vi "CRYGraph Property Window Wave.vi"(9 "Tab Name":string, 10 "Graph VI Ref":refnum<vi>) -> ()   [LabVIEW 2013]
uses:
  <vilib>/Utility/miscctls.llb/LVRowAndColumnTypeDef.ctl
panel:
  in  "SetFormat":bool
  in  "No Data":bool
  out "CursorStyle":string
  out "CursorPointStyle":string
  out "CursorLineWidth":string
  out "CursorLineStyle":string
  out "Scale Style":u8=5
  out "Interpolation":string
  out "PointStyle":string
  out "LineWidth":string
  out "LineStyle":string
  in  "Property Tab":T1(tab)
  in  "Background Color":u32(colorbox)
  in  "Title Name":string
  in  "Ignore timestamp information":bool
  in  "PadType":u16(ring) items=["Pad with spaces on left", "Pad with spaces on right", "Pad with zeros on left"]
  in  "Field Width":u16
  in  "Use minimum field width":bool
  in  "Exponent in multiples of 3":bool
  in  "Hide trailing zeros":bool
  in  "PrecisionDigits":u16
  in  "PrecisionType":u16(ring) items=["Digitals of precision", "Significant digits"]
  in  "Notation":i32(listbox)
  in  "FormatAxis":u16(ring) items=["X-Axis", "Y-Axis"]
  in  "TimeFormat":u16(ring) items=["Custom time format", "System time format", "Time unused"]
  in  "Digits":u16
  in  "YMD":u16(slide)
  in  "AMFM":u16(slide)=1
  in  "HMS":u16(slide)=1
  in  "DateFormat":u16(ring) items=["Custom date format", "System date format", "Date unused"]
  in  "YearShow":u16(slide)
  in  "Point/Fill":u32(colorbox)
  in  "Fill to":i16(ring) items=["none"=-1, "zero"=-2, "-Infinity"=-3, "+Infinity"=-4]
  in  "Items":u16(ring)
  out "Colors":bool
  in  "Line":u32(colorbox)
  in  "LineStyle4":bool
  in  "LineStyle3":bool
  in  "LineStyle2":bool
  in  "LineStyle0":bool
  in  "LineStyle1":bool
  in  "LineWidth5":bool
  in  "LineWidth1":bool
  in  "LineWidth4":bool
  in  "LineWidth3":bool
  in  "LineWidth2":bool
  in  "LineWidth0":bool
  in  "PointStyle16":bool
  in  "PointStyle15":bool
  in  "PointStyle14":bool
  in  "PointStyle13":bool
  in  "PointStyle12":bool
  in  "PointStyle11":bool
  in  "PointStyle10":bool
  in  "PointStyle9":bool
  in  "PointStyle8":bool
  in  "PointStyle7":bool
  in  "PointStyle6":bool
  in  "PointStyle5":bool
  in  "PointStyle4":bool
  in  "PointStyle3":bool
  in  "PointStyle2":bool
  in  "PointStyle1":bool
  in  "PointStyle0":bool
  in  "Interpolation4":bool
  in  "Interpolation5":bool
  in  "Interpolation3":bool
  in  "Interpolation2":bool
  in  "Interpolation1":bool
  in  "Interpolation0":bool
  in  "Show Plot":bool
  in  "GridStyle":u16(ring)=4
  in  "Minor grid":u32(colorbox)
  in  "Major grid":u32(colorbox)
  in  "Marker text":u32(colorbox)
  in  "Minor tick":u32(colorbox)
  in  "Major tick":u32(colorbox)
  in  "Log":bool
  in  "Show scale":bool
  in  "Show scale label":bool
  in  "Maximum":dbl
  in  "Minimum":dbl
  in  "Autoscale":bool
  in  "Axis Name":string caption="Name"
  in  "ScaleAxis":u16(ring)
  out "Grid Colors":bool
  out "Scale Style and Colors":bool
  in  "Cursor Tab":enum32{"Page 1"}(tab)
  in  "CursorPointStyle16":bool
  in  "CursorPointStyle15":bool
  in  "CursorPointStyle14":bool
  in  "CursorPointStyle13":bool
  in  "CursorPointStyle12":bool
  in  "CursorPointStyle11":bool
  in  "CursorPointStyle10":bool
  in  "CursorPointStyle9":bool
  in  "CursorPointStyle8":bool
  in  "CursorPointStyle7":bool
  in  "CursorPointStyle6":bool
  in  "CursorPointStyle5":bool
  in  "CursorPointStyle4":bool
  in  "CursorPointStyle3":bool
  in  "CursorPointStyle2":bool
  in  "CursorPointStyle1":bool
  in  "CursorPointStyle0":bool
  in  "CursorLineWidth5":bool
  in  "CursorLineWidth1":bool
  in  "CursorLineWidth4":bool
  in  "CursorLineWidth3":bool
  in  "CursorLineWidth2":bool
  in  "CursorLineWidth0":bool
  in  "CursorLineStyle4":bool
  in  "CursorLineStyle3":bool
  in  "CursorLineStyle2":bool
  in  "CursorLineStyle0":bool
  in  "CursorLineStyle1":bool
  in  "Cursor Items":u16(ring)
  in  "CursorStyle8":bool
  in  "CursorStyle4":bool
  in  "CursorStyle5":bool
  in  "CursorStyle7":bool
  in  "CursorStyle6":bool
  in  "CursorStyle3":bool
  in  "CursorStyle2":bool
  in  "CursorStyle1":bool
  in  "CursorStyle0":bool
  in  "Cursor color":u32(colorbox)
  in  "Linked to plot:":u16(ring)
  in  "Link Cursors":bool
  in  "Show Cursors":bool
  in  "OK":bool
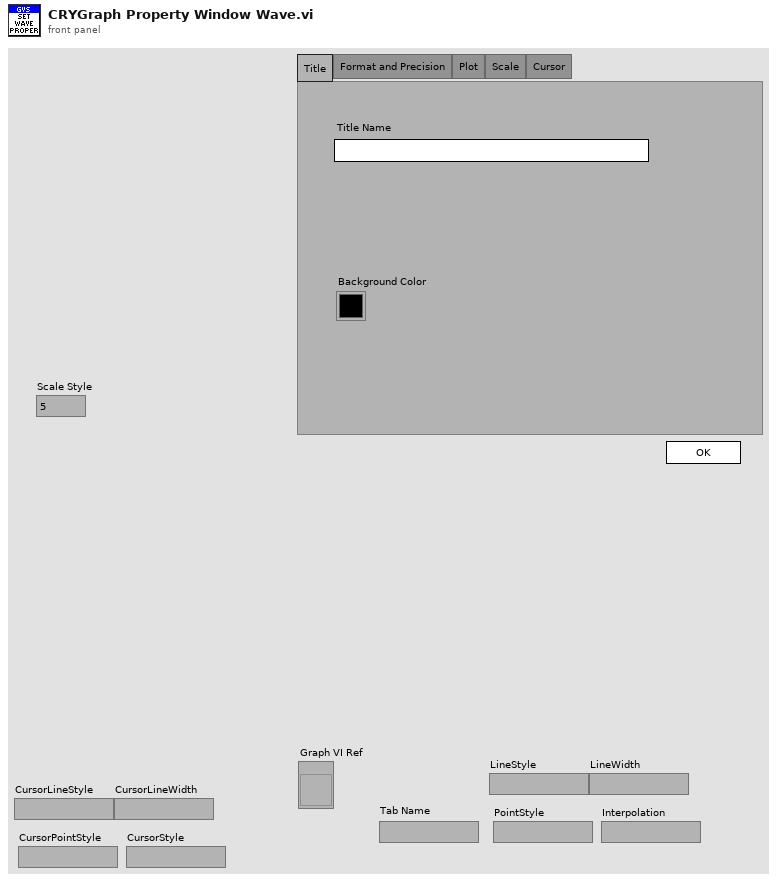
[diagram p1: front panel]
types:
  T1 = enum32{"Title", "Format and Precision", "Plots", "Scales", "Cursors"}
  T2 = enum32{"Page Enabled", "Page Disabled", "Page Disabled & Grayed"}
  T3 = enum8{"Enabled", "Disabled", "Disabled and Grayed Out"}
  T4 = typedef "LVRowAndColumnTypeDef.ctl" = cluster{"Row":i32, "Column":i32}
  T5 = typedef "CRYWaveform Cluster.ctl" = cluster{"Waveform":cluster{"X0":dbl, "dX":dbl, "Y":sgl[]}, "X data":u16, "Y data":u16, "Y axis":u16, "X unit":string, "Y unit":string, "Y dB ref":dbl, "display Y":bool, "display X":bool, "Overload?":bool, "Test Info":string, "Step No.":i32, "Name":string, "protected":bool, "Sqc history":string[], "Signal Channel ID":i32, "Plot Settings":cluster{"Color":u32, "Interpolation":u8, "Point Style":u8, "Line Style":u8, "Point Color":u32, "Line Width":u8, "Bar Plot Style":u8, "Fill To":i16}, "AutoProtect":bool}
  T6 = cluster{"Notation":i32, "PrecisionType":u16, "PrecisionDigits":u16, "Hide trailing zeros":bool, "Exponent in multiples of 3":bool, "Field Width":u16, "PadType":u16, "Use minimum field width":bool, "TimeFormat":u16, "AMFM":u16, "HMS":u16, "Digits":u16, "DateFormat":u16, "YMD":u16, "YearShow":u16}
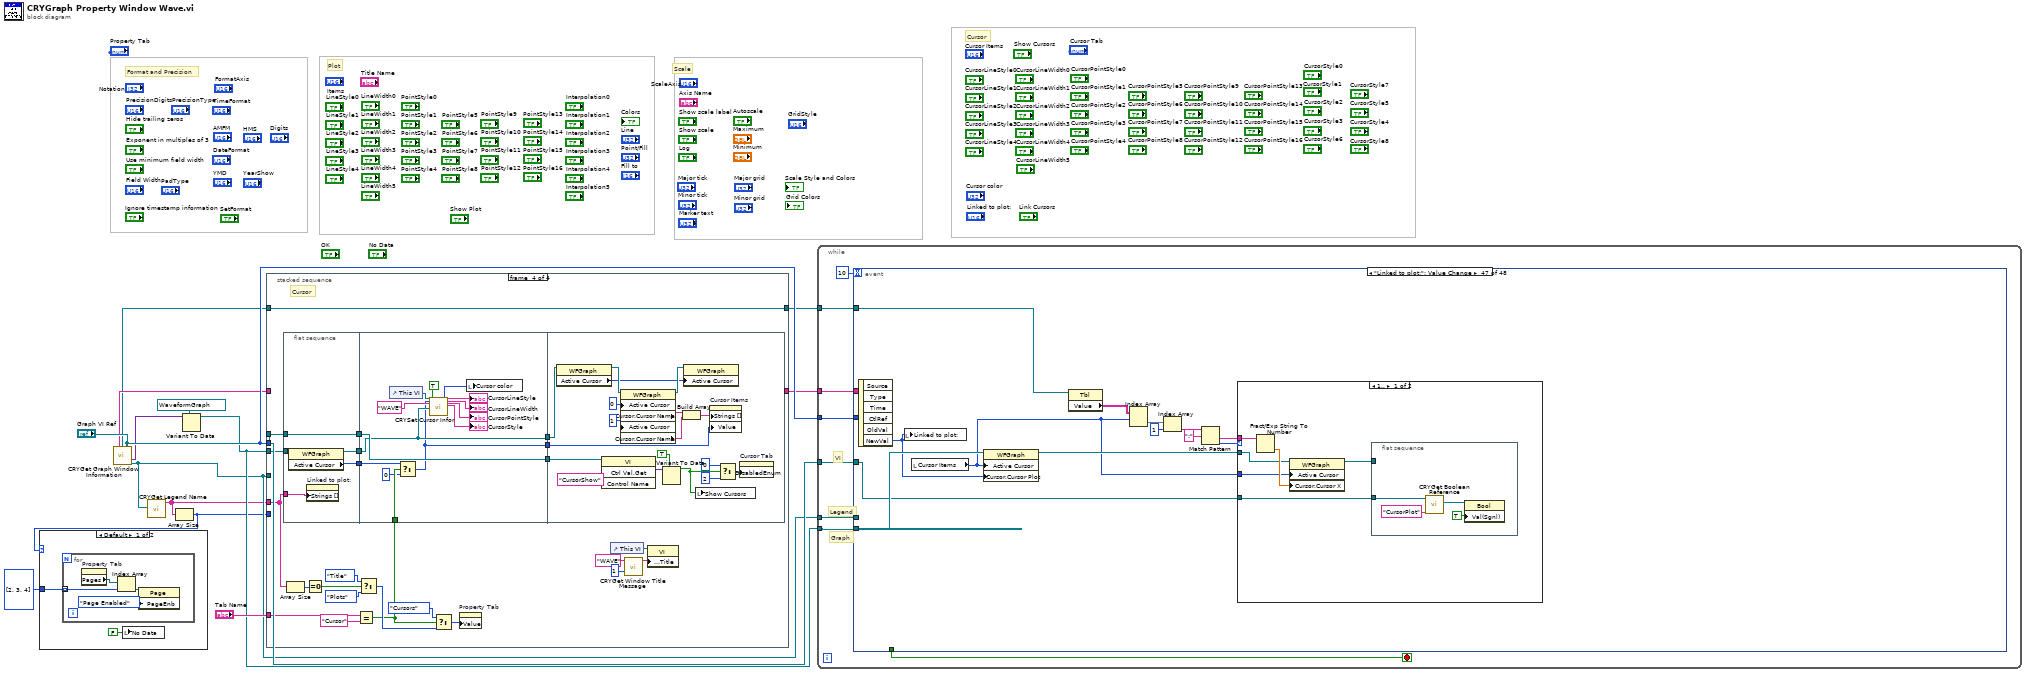
[diagram p0: block diagram]
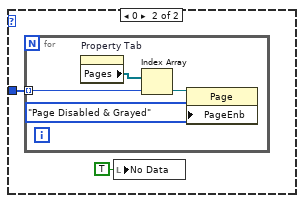
[diagram p2: hidden frame]
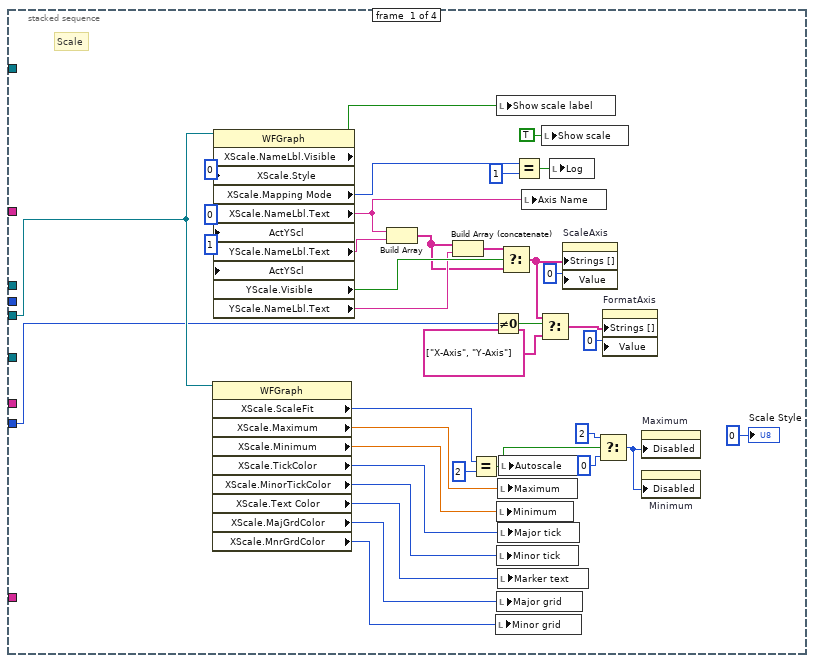
[diagram p3: hidden frame]
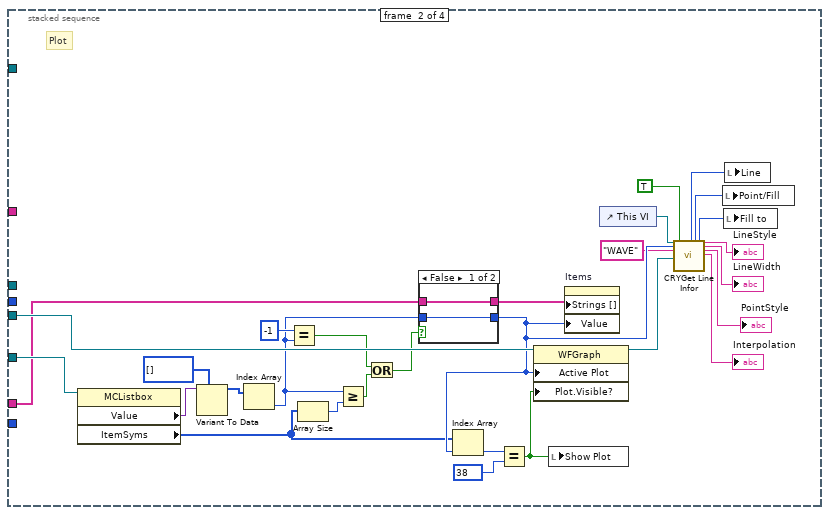
[diagram p4: hidden frame]
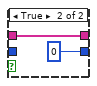
[diagram p5: hidden frame]
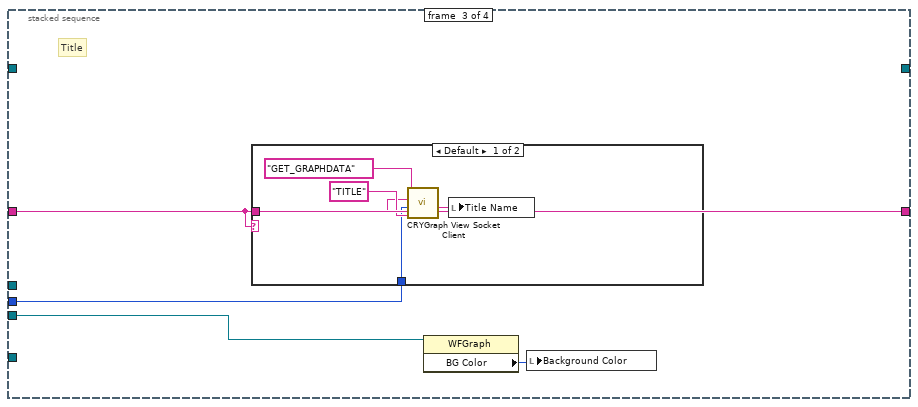
[diagram p6: hidden frame]
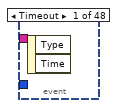
[diagram p8: hidden frame]
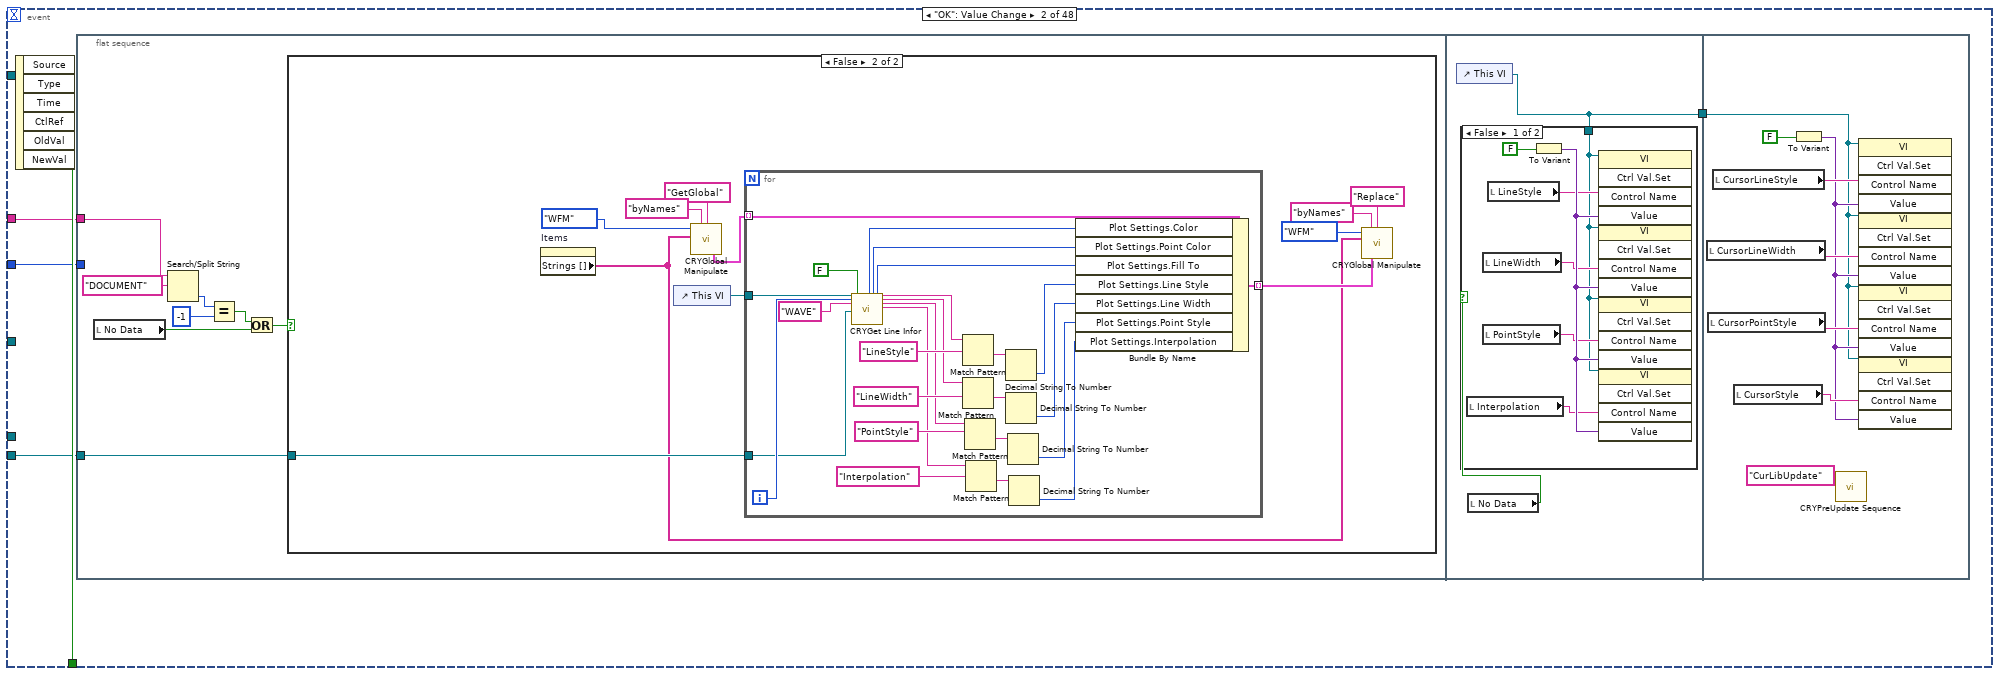
[diagram p9: hidden frame]
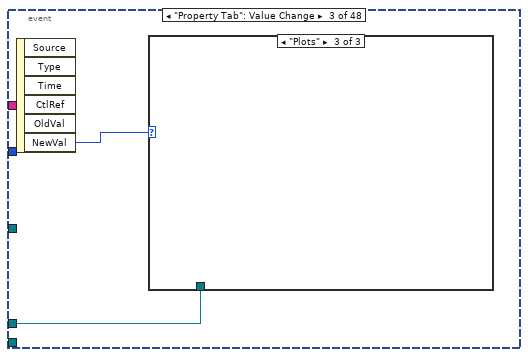
[diagram p12: hidden frame]
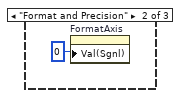
[diagram p14: hidden frame]
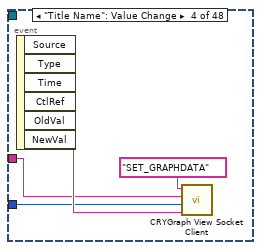
[diagram p15: hidden frame]
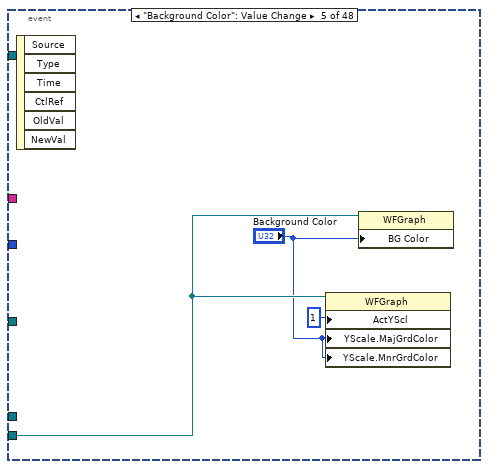
[diagram p16: hidden frame]
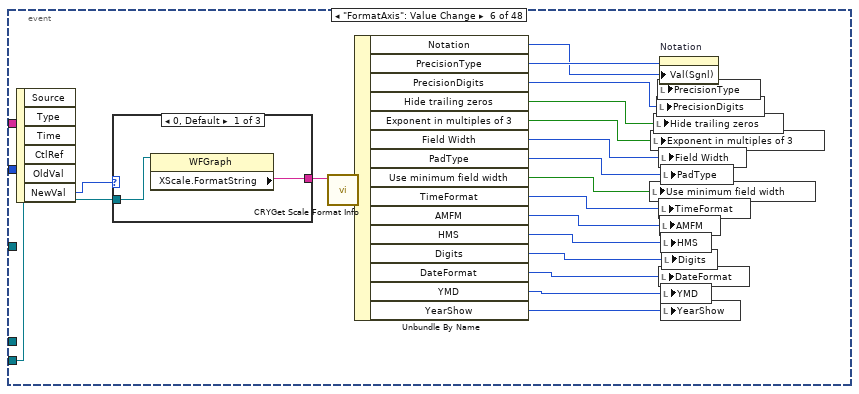
[diagram p17: hidden frame]
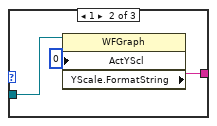
[diagram p18: hidden frame]
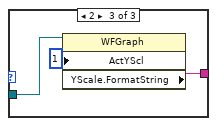
[diagram p19: hidden frame]
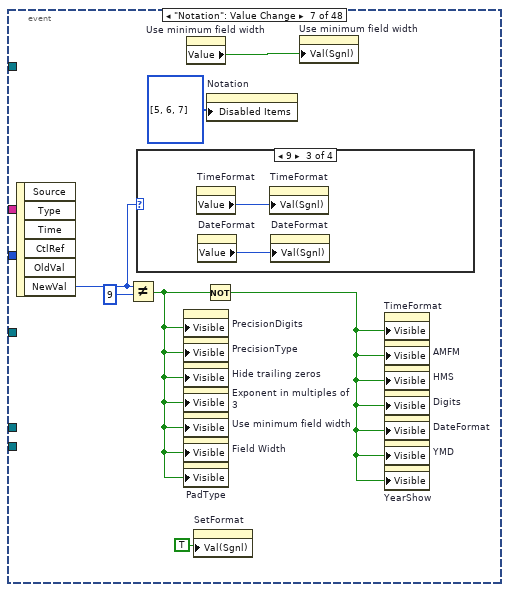
[diagram p20: hidden frame]
diagram:
  # "Format and Precision"
  # "Cursor"
  # "Scale"
  # "Plot"
  n1 = call "CRYGet Graph Window Information.vi"("pGraph VI In"="Graph VI Ref") -> ("Queue Name Out"=w10:string, "Cursor Ref Out"=w2:refnum<vi>, "Graph Number Out"=w11:i32, "Graph Control Ref Out"=w4:variant, "Legend Ref Out"=w8:refnum<vi>)  [unwired: 2 in, 8 out]
  n2 = call "CRYGet Legend Name.vi"("MCListbox Refnum"=w8) -> ("Names Out"=w7:string[])  [unwired: 1 in, 9 out]
  n3 = Array Size(array=w7) -> (size(s)=w6:i32)
  n4 = case shown="Default" w6 {
    tunnel: i32[] [2, 3, 4] -> [w15 w21]
    frame Default {
      n5 = for {
        tunnel: w15 -> [w18] mode=indexing
        n6 = property on="Property Tab" class="TabCtl (strict)"() -> ("Pages"=w17:refnum<vi>[])  [unwired: 2 in, 2 out]
        n7 = Index Array(array=w17, index=w18) -> (element=w19:refnum<vi>)
        n8 = property class="Page"(reference=w19, "PageEnb"=T2."Page Enabled" ("Page Enabled State")) -> ()  [unwired: 1 in, 2 out]
      }
      n9 = local write "No Data"(FALSE ("No Data")) -> ()
    }
    frame 0 {
      n10 = for {
        tunnel: w21 -> [w23] mode=indexing
        n11 = property on="Property Tab" class="TabCtl (strict)"() -> ("Pages"=w24:refnum<vi>[])  [unwired: 2 in, 2 out]
        n12 = Index Array(array=w24, index=w23) -> (element=w25:refnum<vi>)
        n13 = property class="Page"(reference=w25, "PageEnb"=T2."Page Disabled & Grayed" ("Page Enabled State")) -> ()  [unwired: 1 in, 2 out]
      }
      n14 = local write "No Data"(TRUE ("No Data")) -> ()
    }
  }
  n15 = Variant To Data(type=refnum<vi> refnum ("WaveGraph Ref"), Variant=w4) -> (data=w12:refnum<vi>)  [unwired: 1 in, 1 out]
  n16 = stacked-sequence {
    tunnel: w12 -> [w62 w90 w99 w128]
    tunnel: "Graph VI Ref" -> [_ _ _ w125]
    tunnel: w8 -> [_ w91 _ _]
    tunnel: "Tab Name" -> [_ _ _ w120]
    tunnel: w11 -> [_ _ w97 _]
    tunnel: w10 -> [_ _ w96 _]
    tunnel: [_ _ w96 _] -> w9
    tunnel: w7 -> [_ w89 _ w117]
    tunnel: w6 -> [w30 _ _ _]
    tunnel: w2 -> [_ _ _ w105]
    tunnel: [_ _ _ w105] -> w1
    frame #0 {
      # "Scale"
      n17 = property class="WFGraph"(reference=w62) -> ("XScale.ScaleFit"=w52:u8, "XScale.Maximum"=w51:dbl, "XScale.Minimum"=w50:dbl, "XScale.TickColor"=w43:u32, "XScale.MinorTickColor"=w42:u32, "XScale.Text Color"=w41:u32, "XScale.MajGrdColor"=w40:u32, "XScale.MnrGrdColor"=w39:u32)  [unwired: 1 in, 2 out]
      n18 = property class="WFGraph"(reference=w62, "XScale.Style"=u8 0 ("X Scale.Style"), "ActYScl"=0 ("Active Y Scale"), "ActYScl"=1 ("Active Y Scale")) -> ("XScale.NameLbl.Visible"=w59:bool, "XScale.Mapping Mode"=w55:u8, "XScale.NameLbl.Text"=w44:string, "YScale.NameLbl.Text"=w38:string, "YScale.Visible"=w36:bool, "YScale.NameLbl.Text"=w35:string)  [unwired: 1 in, 2 out]
      n19 = Build Array(w44, w38) -> (w33:string[])
      n20 = Build Array (concatenate)(w33, w35) -> (w34:string[])
      n21 = Equal?(x=w52, y=u8 2 ("X Scale.Scale Fit")) -> (x = y?=w45:bool)
      n22 = Not Equal To 0?(x=w30) -> (x != 0?=w31:bool)
      n23 = local write "Minor grid"(w39) -> ()
      n24 = local write "Show scale label"(w59) -> ()
      n25 = local write "Minimum"(w50) -> ()
      n26 = local write "Minor tick"(w42) -> ()
      n27 = local write "Major grid"(w40) -> ()
      n28 = local write "Maximum"(w51) -> ()
      n29 = local write "Major tick"(w43) -> ()
      n30 = local write "Marker text"(w41) -> ()
      n31 = local write "Autoscale"(w45) -> ()
      n32 = Select(t=w34, s=w36, f=w33) -> (s? t:f=w29:string[])
      n33 = Equal?(x=w55, y=u8 1) -> (x = y?=w56:bool)
      n34 = local write "Axis Name"(w44) -> ()
      n35 = Select(t=w29, s=w31, f=string[] ["X-Axis", "Y-Axis"]) -> (s? t:f=w28:string[])
      n36 = local write "Show scale"(TRUE ("Show scale")) -> ()
      n37 = local write "Log"(w56) -> ()
      n38 = property on="ScaleAxis" class="Ring (strict)"("Strings []"=w29, "Value"=u8 0 ("y")) -> ()  [unwired: 2 in, 2 out]
      n39 = Select(t=u8 2 ("X Scale.Scale Fit"), s=w45, f=u8 0 ("X Scale.Scale Fit")) -> (s? t:f=w47:u8)
      n40 = property on="FormatAxis" class="Ring (strict)"("Strings []"=w28, "Value"=u8 0 ("y")) -> ()  [unwired: 2 in, 2 out]
      n41 = property on="Maximum" class="DigNum (strict)"("Disabled"=w47) -> ()  [unwired: 2 in, 2 out]
      n42 = property on="Minimum" class="DigNum (strict)"("Disabled"=w47) -> ()  [unwired: 2 in, 2 out]
      "Scale Style" <- u8 0 ("X Scale.Scale Fit")
    }
    frame #1 {
      # "Plot"
      n43 = property class="MCListbox"(reference=w91) -> ("Value"=w83:variant, "ItemSyms"=w69:i32[])  [unwired: 1 in, 2 out]
      n44 = Variant To Data(type=i32[] [], Variant=w83) -> (data=w70:i32[])  [unwired: 1 in, 1 out]
      n45 = Index Array(array=w70) -> (element=w63:i32)  [unwired: 1 in]
      n46 = Equal?(x=-1, y=w63) -> (x = y?=w66:bool)
      n47 = Array Size(array=w69) -> (size(s)=w67:i32)
      n48 = Greater Or Equal?(x=w63, y=w67) -> (x >= y?=w65:bool)
      n49 = Or(x=w66, y=w65) -> (x .or. y?=w64:bool)
      n50 = case shown="False" w64 {
        tunnel: w89 -> [w93 w95]
        tunnel: [w93 w95] -> w88
        tunnel: [w92 0 ("Value")] -> w82
        tunnel: w63 -> [w92 _]
        frame False {
        }
        frame True {
        }
      }
      n51 = Index Array(array=w69, index=w82) -> (element=w86:i32)
      n52 = Equal?(x=w86, y=38) -> (x = y?=w84:bool)
      n53 = property class="WFGraph"(reference=w90, "Active Plot"=w82, "Plot.Visible?"=w84) -> (reference out=w87:refnum<vi>)  [unwired: 1 in, 1 out]
      n54 = local write "Show Plot"(w84) -> ()
      n55 = property on="Items" class="Ring (strict)"("Strings []"=w88, "Value"=w82) -> ()  [unwired: 2 in, 2 out]
      n56 = control-ref of="This VI"() -> (w77:refnum<vi>)
      n57 = call "CRYGet Line Infor.vi"("This VI"=w77, "Active Plot Number"=w82, "Graph Type"="WAVE", "Wave Graph Control Ref"=w87, "Property Set?"=TRUE) -> ("Line"=w73:u32, "Point/Fill"=w72:u32, "Fill to"=w74:i16, "LineStyle"=→"LineStyle":string, "LineWidth"=→"LineWidth":string, "PointStyle"=→"PointStyle":string, "Interpolation"=→"Interpolation":string)  [unwired: 16 in]
      n58 = local write "Point/Fill"(w72) -> ()
      n59 = local write "Fill to"(w74) -> ()
      n60 = local write "Line"(w73) -> ()
    }
    frame #2 {
      # "Title"
      n61 = case shown="Default" w96 {
        tunnel: w97 -> [w102 _]
        tunnel: w96 -> [w101 _]
        frame Default {
          n62 = call "CRYGraph View Socket Client.vi"("sOption"="TITLE", "nData"=w102, "sData"=w101, "sAction"="GET_GRAPHDATA") -> ("sData Out"=w100:string)  [unwired: 4 in, 3 out]
          n63 = local write "Title Name"(w100) -> ()
        }
        frame "test DataView" {
        }
      }
      n64 = property class="WFGraph"(reference=w99) -> ("BG Color"=w98:u32)  [unwired: 1 in, 2 out]
      n65 = local write "Background Color"(w98) -> ()
    }
    frame #3 {
      # "Cursor"
      n66 = flat-sequence {
        tunnel: w125 -> [w133]
        tunnel: w128 -> [w131]
        tunnel: [w130] -> w119
        tunnel: [w133] -> w118
        tunnel: w117 -> [w132]
        tunnel: [w129] -> w115
        tunnel: [w136] -> w127
        tunnel: [w139] -> w126
        tunnel: w119 -> [w136]
        tunnel: w118 -> [w139]
        tunnel: w116 -> [w138]
        tunnel: w115 -> [w135]
        tunnel: [w134] -> w114
        tunnel: w127 -> [w152]
        tunnel: w126 -> [w153]
        tunnel: w114 -> [w148]
        frame #0 {
          n67 = property class="WFGraph"(reference=w131) -> (reference out=w130:refnum<vi>, "Active Cursor"=w129:u32)  [unwired: 1 in, 1 out]
          n68 = property on="Linked to plot:" class="Ring (strict)"("Strings []"=w132) -> ()  [unwired: 2 in, 2 out]
        }
        frame #1 {
          n69 = control-ref of="This VI"() -> (w140:refnum<vi>)
          n70 = Select(t=w135, s=w138, f=u32 0 ("Active Cursor")) -> (s? t:f=w134:u32)
          n71 = call "CRYSet Cursor Infor.vi"("This VI"=w140, "Active Cursor"=w134, "Graph Type"="WAVE", "Wave Graph Ref"=w136, "Property Set?"=TRUE) -> ("Cursor Color"=w147:u32, "CursorLineStyle"=→"CursorLineStyle":string, "CursorLineWidth"=→"CursorLineWidth":string, "CursorPointStyle"=→"CursorPointStyle":string, "CursorStyle"=→"CursorStyle":string)  [unwired: 17 in, 1 out]
          n72 = local write "Cursor color"(w147) -> ()
        }
        frame #2 {
          n73 = property class="WFGraph"(reference=w152) -> (reference out=w151:refnum<vi>, "Active Cursor"=w149:u32)  [unwired: 1 in, 1 out]
          n74 = invoke class="VI" method="Ctrl Val.Get"(reference=w153, "Control Name"="CursorShow") -> ("Get Control Value Variant"=w158:variant)  [unwired: 2 in, 3 out]
          n75 = property class="WFGraph"(reference=w151, "Active Cursor"=u32 0, "Active Cursor"=u32 1) -> (reference out=w150:refnum<vi>, "Cursor.Cursor Name"=w163:string, "Cursor.Cursor Name"=w162:string)  [unwired: 1 in, 1 out]
          n76 = Variant To Data(type=TRUE ("Visible"), Variant=w158) -> (data=w160:bool)  [unwired: 1 in, 1 out]
          n77 = Build Array(w163, w162) -> (w161:string[])
          n78 = property class="WFGraph"(reference=w150, "Active Cursor"=w149) -> ()  [unwired: 1 in, 2 out]
          n79 = local write "Show Cursors"(w160) -> ()
          n80 = property on="Cursor Items" class="Ring (strict)"("Strings []"=w161, "Value"=w148) -> ()  [unwired: 2 in, 2 out]
          n81 = Select(t=0, s=w160, f=2) -> (s? t:f=w156:i32)
          n82 = property on="Cursor Tab" class="TabCtl (strict)"("DisabledEnum"=w156) -> ()  [unwired: 2 in, 2 out]
        }
      }
      n83 = Array Size(array=w117) -> (size(s)=w124:i32)
      n84 = Equal To 0?(x=w124) -> (x = 0?=w122:bool)
      n85 = Equal?(x=w120, y="Cursor" ("Graph Type")) -> (x = y?=w116:bool)
      n86 = Select(t=T1."Title" ("Tab Control"), s=w122, f=T1."Plots" ("Tab Control")) -> (s? t:f=w121:T1)
      n87 = Select(t=T1."Cursors" ("Tab Control"), s=w116, f=w121) -> (s? t:f=w110:T1)
      n88 = property on="Property Tab" class="TabCtl (strict)"("Value"=w110) -> ()  [unwired: 2 in, 2 out]
      n89 = control-ref of="This VI"() -> (w106:refnum<vi>)
      n90 = call "CRYGet Window Title Message.vi"("No"=1 ("Error No"), "Kind"="WAVE") -> ("Multibyte String"=w107:string)  [unwired: 4 in, 5 out]
      n91 = property class="VI"(reference=w106, "Front Panel.Title"=w107) -> ()  [unwired: 1 in, 2 out]
    }
  }
  n92 = while {
    tunnel: w12 -> [w172]
    tunnel: "Graph VI Ref" -> [w171]
    tunnel: w8 -> [w169]
    tunnel: w9 -> [w168]
    tunnel: w11 -> [w167]
    tunnel: w1 -> [w166]
    stop <- w173 stop-if-true
    # "Legend"
    # "Graph"
    # "VI"
    n93 = event shown="[46] \"Linked to plot:\": Value Change" {
      selector: _ -> [_ _ _ _ _ _ _ _ _ _ _ _ _ _ _ _ _ _ _ _ _ _ _ _ _ _ _ _ _ _ _ _ _ _ _ _ _ _ _ _ _ _ _ _ _ _ _ _]
      dyn-events: _ -> [_ _ _ _ _ _ _ _ _ _ _ _ _ _ _ _ _ _ _ _ _ _ _ _ _ _ _ _ _ _ _ _ _ _ _ _ _ _ _ _ _ _ _ _ _ _ _ _]
      timeout: 10 -> [_ _ _ _ _ _ _ _ _ _ _ _ _ _ _ _ _ _ _ _ _ _ _ _ _ _ _ _ _ _ _ _ _ _ _ _ _ _ _ _ _ _ _ _ _ _ _ _]
      tunnel: [_ w178 _ _ _ _ _ _ _ _ _ _ _ _ _ _ _ _ _ _ _ _ _ _ _ _ _ _ _ _ _ _ _ _ _ _ _ _ _ _ _ _ _ _ _ _ _ _] -> w173
      tunnel: w172 -> [_ w177 _ _ w249 w268 _ _ _ _ _ _ _ _ _ w337 w481 w513 w545 w577 w607 w640 w656 w666 w676 w704 w746 w757 w770 w786 w800 w811 w822 w833 w844 w855 w872 w928 w947 _ w971 w992 w1013 w1034 w1055 w1078 w1098 _]
      tunnel: w171 -> [_ _ _ _ _ _ _ _ _ _ _ _ _ _ _ _ _ _ _ _ _ _ _ _ _ _ _ _ _ _ _ _ _ _ _ _ w868 w925 w944 w966 _ _ _ _ _ w1079 w1086 _]
      tunnel: w169 -> [_ _ w241 _ _ _ _ _ _ _ _ _ _ _ _ _ w479 w511 w543 w575 w609 w639 w655 w663 w674 _ _ _ _ _ _ _ _ _ _ _ _ _ _ _ _ _ _ _ _ _ _ _]
      tunnel: w168 -> [_ w175 _ w245 _ _ _ _ _ _ _ _ _ _ _ _ w480 w512 w544 w576 _ _ w650 w664 w673 _ _ _ _ _ _ _ _ _ _ _ _ _ _ _ _ _ _ _ _ _ _ _]
      tunnel: w167 -> [_ w174 _ w244 _ _ _ _ _ _ _ _ _ _ _ _ _ _ _ _ _ _ _ _ _ _ _ _ _ _ _ _ _ _ _ _ _ _ _ _ _ _ _ _ _ _ _ _]
      tunnel: w166 -> [_ _ _ _ _ _ _ _ _ _ _ _ _ _ _ _ _ _ _ _ _ _ _ _ _ _ _ _ _ _ _ _ _ _ _ _ _ _ _ _ _ _ _ _ _ _ w1087 _]
      event Timeout {
        n94 = event-data() -> ()  [unwired: 3 out]
      }
      event "OK": Value Change {
        n95 = event-data() -> ("NewVal"=w178:bool)  [unwired: 6 out]
        n96 = flat-sequence {
          tunnel: w177 -> [w186]
          tunnel: w175 -> [w179]
          tunnel: w174 -> [_]
          tunnel: [w225] -> w176
          tunnel: w176 -> [w234]
          frame #0 {
            n97 = local read "No Data"() -> (w181:bool)
            n98 = Search/Split String(string=w179, search string/char (-)="DOCUMENT" ("regular expression")) -> (offset of match=w184:i32)  [unwired: 1 in, 2 out]
            n99 = Equal?(x=w184, y=-1) -> (x = y?=w182:bool)
            n100 = Or(x=w182, y=w181) -> (x .or. y?=w180:bool)
            n101 = case shown="False" w180 {
              tunnel: w186 -> [_ w197]
              frame True {
              }
              frame False {
                n102 = property on="Items" class="Ring (strict)"() -> ("Strings []"=w188:string[])  [unwired: 2 in, 2 out]
                n103 = control-ref of="This VI"() -> (w196:refnum<vi>)
                n104 = call "CRYGlobal Manipulate.vi"("Type"=enum16{"Curves", "Values", "Results", "WFM"}."WFM" ("Type In"), "sOption"="byNames", "sAction"="GetGlobal", "sData"=w188) -> ("WFM Out"=w194:T5[])  [unwired: 5 in, 6 out]
                n105 = for {
                  tunnel: w196 -> [w222]
                  tunnel: w197 -> [w204]
                  tunnel: [w199] -> w193 mode=indexing
                  tunnel: w194 -> [w198] mode=indexing
                  i -> [w206]
                  n106 = call "CRYGet Line Infor.vi"("This VI"=w222, "Active Plot Number"=w206, "Graph Type"="WAVE", "Wave Graph Control Ref"=w204, "Property Set?"=FALSE) -> ("Line"=w201:u32, "Point/Fill"=w200:u32, "Fill to"=w202:i16, "LineStyle"=w213:string, "LineWidth"=w209:string, "PointStyle"=w208:string, "Interpolation"=w207:string)  [unwired: 16 in]
                  n107 = Match Pattern(string=w213, regular expression="LineStyle") -> (after substring=w219:string)  [unwired: 4 out]
                  n108 = Match Pattern(string=w209, regular expression="LineWidth") -> (after substring=w220:string)  [unwired: 4 out]
                  n109 = Match Pattern(string=w208, regular expression="PointStyle") -> (after substring=w218:string)  [unwired: 4 out]
                  n110 = Match Pattern(string=w207, regular expression="Interpolation") -> (after substring=w215:string)  [unwired: 4 out]
                  n111 = Decimal String To Number(string=w219) -> (number=w212:i32)  [unwired: 3 out]
                  n112 = Decimal String To Number(string=w220) -> (number=w211:i32)  [unwired: 3 out]
                  n113 = Decimal String To Number(string=w218) -> (number=w210:i32)  [unwired: 3 out]
                  n114 = Decimal String To Number(string=w215) -> (number=w205:i32)  [unwired: 3 out]
                  n115 = Bundle By Name(cluster=w198, "Plot Settings.Color"=w201, "Plot Settings.Point Color"=w200, "Plot Settings.Fill To"=w202, "Plot Settings.Line Style"=w212, "Plot Settings.Line Width"=w211, "Plot Settings.Point Style"=w210, "Plot Settings.Interpolation"=w205) -> (w199:T5)
                }
                n116 = call "CRYGlobal Manipulate.vi"("Type"=enum16{"Curves", "Values", "Results", "WFM"}."WFM", "sOption"="byNames", "sAction"="Replace", "sData"=w188, "WFM"=w193) -> ()  [unwired: 4 in, 7 out]
              }
            }
          }
          frame #1 {
            n117 = control-ref of="This VI"() -> (w225:refnum<vi>)
            n118 = local read "No Data"() -> (w224:bool)
            n119 = case shown="False" w224 {
              tunnel: w225 -> [w226 _]
              frame False {
                n120 = local read "Interpolation"() -> (w227:string)
                n121 = local read "LineWidth"() -> (w229:string)
                n122 = local read "PointStyle"() -> (w228:string)
                n123 = local read "LineStyle"() -> (w230:string)
                n124 = To Variant(anything=FALSE) -> (Variant=w232:variant)
                n125 = invoke class="VI" method="Ctrl Val.Set"(reference=w226, "Control Name"=w230, "Value"=w232) -> ()  [unwired: 2 in, 5 out]
                n126 = invoke class="VI" method="Ctrl Val.Set"(reference=w226, "Control Name"=w229, "Value"=w232) -> ()  [unwired: 2 in, 5 out]
                n127 = invoke class="VI" method="Ctrl Val.Set"(reference=w226, "Control Name"=w228, "Value"=w232) -> ()  [unwired: 2 in, 5 out]
                n128 = invoke class="VI" method="Ctrl Val.Set"(reference=w226, "Control Name"=w227, "Value"=w232) -> ()  [unwired: 2 in, 5 out]
              }
              frame True {
              }
            }
          }
          frame #2 {
            n129 = local read "CursorLineWidth"() -> (w238:string)
            n130 = local read "CursorPointStyle"() -> (w239:string)
            n131 = local read "CursorLineStyle"() -> (w237:string)
            n132 = local read "CursorStyle"() -> (w240:string)
            n133 = To Variant(anything=FALSE) -> (Variant=w235:variant)
            n134 = call "CRYPreUpdate Sequence.vi"("EventName"="CurLibUpdate") -> ()  [unwired: 15 in]
            n135 = invoke class="VI" method="Ctrl Val.Set"(reference=w234, "Control Name"=w237, "Value"=w235) -> ()  [unwired: 2 in, 5 out]
            n136 = invoke class="VI" method="Ctrl Val.Set"(reference=w234, "Control Name"=w238, "Value"=w235) -> ()  [unwired: 2 in, 5 out]
            n137 = invoke class="VI" method="Ctrl Val.Set"(reference=w234, "Control Name"=w239, "Value"=w235) -> ()  [unwired: 2 in, 5 out]
            n138 = invoke class="VI" method="Ctrl Val.Set"(reference=w234, "Control Name"=w240, "Value"=w235) -> ()  [unwired: 2 in, 5 out]
          }
        }
      }
      event "Property Tab": Value Change {
        n139 = event-data() -> ("NewVal"=w242:T1)  [unwired: 6 out]
        n140 = case shown="\"Plots\"" w242 {
          tunnel: w241 -> [_ _ _]
          frame "Title", Default {
          }
          frame "Format and Precision" {
            n141 = property on="FormatAxis" class="Ring (strict)"("Val(Sgnl)"=0 ("Value (Signaling)")) -> ()  [unwired: 2 in, 2 out]
          }
          frame "Plots" {
          }
        }
      }
      event "Title Name": Value Change {
        n142 = event-data() -> ("NewVal"=w246:string)  [unwired: 6 out]
        n143 = call "CRYGraph View Socket Client.vi"("sOption"=w246, "nData"=w244, "sData"=w245, "sAction"="SET_GRAPHDATA") -> ()  [unwired: 4 in, 4 out]
      }
      event "Background Color": Value Change {
        n144 = event-data() -> ()  [unwired: 7 out]
        n145 = property on="Property Node" class="WFGraph"(reference=w249, "ActYScl"=1 ("Active Y Scale"), "YScale.MajGrdColor"="Background Color", "YScale.MnrGrdColor"="Background Color") -> ()  [unwired: 1 in, 2 out]
        n146 = property class="WFGraph"(reference=w249, "BG Color"="Background Color") -> ()  [unwired: 1 in, 2 out]
      }
      event "FormatAxis": Value Change {
        n147 = event-data() -> ("NewVal"=w269:u16)  [unwired: 6 out]
        n148 = case shown="0, Default" w269 {
          tunnel: w268 -> [w271 w274 w277]
          tunnel: [w270 w272 w275] -> w267
          frame 0, Default {
            n149 = property class="WFGraph"(reference=w271) -> ("XScale.FormatString"=w270:string)  [unwired: 1 in, 2 out]
          }
          frame 1 {
            n150 = property class="WFGraph"(reference=w274, "ActYScl"=0 ("Active Y Scale")) -> ("YScale.FormatString"=w272:string)  [unwired: 1 in, 2 out]
          }
          frame 2 {
            n151 = property class="WFGraph"(reference=w277, "ActYScl"=1 ("Active Y Scale")) -> ("YScale.FormatString"=w275:string)  [unwired: 1 in, 2 out]
          }
        }
        n152 = call "CRYGet Scale Format Info.vi"("FormatString"=w267) -> ("ScaleFormat"=w266:T6)  [unwired: 10 in]
        n153 = Unbundle By Name(w266) -> ("Notation"=w259:i32, "PrecisionType"=w265:u16, "PrecisionDigits"=w264:u16, "Hide trailing zeros"=w263:bool, "Exponent in multiples of 3"=w262:bool, "Field Width"=w261:u16, "PadType"=w260:u16, "Use minimum field width"=w258:bool, "TimeFormat"=w257:u16, "AMFM"=w256:u16, "HMS"=w255:u16, "Digits"=w254:u16, "DateFormat"=w253:u16, "YMD"=w252:u16, "YearShow"=w251:u16)
        n154 = local write "Use minimum field width"(w258) -> ()
        n155 = local write "Exponent in multiples of 3"(w262) -> ()
        n156 = local write "Hide trailing zeros"(w263) -> ()
        n157 = local write "PrecisionDigits"(w264) -> ()
        n158 = local write "PrecisionType"(w265) -> ()
        n159 = local write "Field Width"(w261) -> ()
        n160 = local write "TimeFormat"(w257) -> ()
        n161 = local write "DateFormat"(w253) -> ()
        n162 = property on="Notation" class="LstBox (strict)"("Val(Sgnl)"=w259) -> ()  [unwired: 2 in, 2 out]
        n163 = local write "AMFM"(w256) -> ()
        n164 = local write "PadType"(w260) -> ()
        n165 = local write "HMS"(w255) -> ()
        n166 = local write "YMD"(w252) -> ()
        n167 = local write "YearShow"(w251) -> ()
        n168 = local write "Digits"(w254) -> ()
      }
      event "Notation": Value Change {
        n169 = event-data() -> ("NewVal"=w283:i32)  [unwired: 6 out]
        n170 = Not Equal?(x=w283, y=9) -> (x != y?=w281:bool)
        n171 = case shown="9" w283 {
          frame 0, 3 {
            n172 = property on="Exponent in multiples of 3" class="Bool (strict)"("DisabledEnum"=T3."Enabled" ("Disabled")) -> ()  [unwired: 2 in, 2 out]
          }
          frame 1, 2 {
            n173 = property on="Exponent in multiples of 3" class="Bool (strict)"("DisabledEnum"=T3."Disabled and Grayed Out" ("Disabled")) -> ()  [unwired: 2 in, 2 out]
          }
          frame 9 {
            n174 = property on="TimeFormat" class="Ring (strict)"() -> ("Value"=w288:u16)  [unwired: 2 in, 2 out]
            n175 = property on="DateFormat" class="Ring (strict)"() -> ("Value"=w287:u16)  [unwired: 2 in, 2 out]
            n176 = property on="TimeFormat" class="Ring (strict)"("Val(Sgnl)"=w288) -> ()  [unwired: 2 in, 2 out]
            n177 = property on="DateFormat" class="Ring (strict)"("Val(Sgnl)"=w287) -> ()  [unwired: 2 in, 2 out]
          }
          frame Default {
          }
        }
        n178 = property on="PrecisionDigits" class="DigNum (strict)"("Visible"=w281) -> ()  [unwired: 2 in, 2 out]
        n179 = property on="PrecisionType" class="Ring (strict)"("Visible"=w281) -> ()  [unwired: 2 in, 2 out]
        n180 = property on="Hide trailing zeros" class="Bool (strict)"("Visible"=w281) -> ()  [unwired: 2 in, 2 out]
        n181 = property on="Exponent in multiples of 3" class="Bool (strict)"("Visible"=w281) -> ()  [unwired: 2 in, 2 out]
        n182 = property on="Use minimum field width" class="Bool (strict)"("Visible"=w281) -> ()  [unwired: 2 in, 2 out]
        n183 = property on="Field Width" class="DigNum (strict)"("Visible"=w281) -> ()  [unwired: 2 in, 2 out]
        n184 = property on="PadType" class="Ring (strict)"("Visible"=w281) -> ()  [unwired: 2 in, 2 out]
        n185 = property on="Use minimum field width" class="Bool (strict)"() -> ("Value"=w278:bool)  [unwired: 2 in, 2 out]
        n186 = property on="SetFormat" class="Bool (strict)"("Val(Sgnl)"=TRUE ("Value (Signaling)")) -> ()  [unwired: 2 in, 2 out]
        n187 = Not(x=w281) -> (.not. x?=w280:bool)
        n188 = property on="Notation" class="LstBox (strict)"("Disabled Items"=i32[] [5, 6, 7]) -> ()  [unwired: 2 in, 2 out]
        n189 = property on="Use minimum field width" class="Bool (strict)"("Val(Sgnl)"=w278) -> ()  [unwired: 2 in, 2 out]
        n190 = property on="TimeFormat" class="Ring (strict)"("Visible"=w280) -> ()  [unwired: 2 in, 2 out]
        n191 = property on="AMFM" class="Slide (strict)"("Visible"=w280) -> ()  [unwired: 2 in, 2 out]
        n192 = property on="HMS" class="Slide (strict)"("Visible"=w280) -> ()  [unwired: 2 in, 2 out]
        n193 = property on="Digits" class="DigNum (strict)"("Visible"=w280) -> ()  [unwired: 2 in, 2 out]
        n194 = property on="DateFormat" class="Ring (strict)"("Visible"=w280) -> ()  [unwired: 2 in, 2 out]
        n195 = property on="YMD" class="Slide (strict)"("Visible"=w280) -> ()  [unwired: 2 in, 2 out]
        n196 = property on="YearShow" class="Slide (strict)"("Visible"=w280) -> ()  [unwired: 2 in, 2 out]
      }
      event "PrecisionType", "PrecisionDigits", "Hide trailing zeros", "Exponent in multiples of 3", "PadType": Value Change {
        n197 = event-data() -> ()  [unwired: 7 out]
        n198 = property on="SetFormat" class="Bool (strict)"("Val(Sgnl)"=TRUE ("Value (Signaling)")) -> ()  [unwired: 2 in, 2 out]
      }
      event "Use minimum field width": Value Change {
        n199 = event-data() -> ("NewVal"=w298:bool)  [unwired: 6 out]
        n200 = property on="Field Width" class="DigNum (strict)"() -> ("Value"=w291:u16)  [unwired: 2 in, 2 out]
        n201 = Equal To 0?(x=w291) -> (x = 0?=w293:bool)
        n202 = Select(t=u16 1 ("Field Width"), s=w293, f=w291) -> (s? t:f=w290:u16)
        n203 = Select(t=T3."Enabled" ("Disabled"), s=w298, f=T3."Disabled and Grayed Out") -> (s? t:f=w299:T3)
        n204 = Select(t=w290, s=w298, f=u16 0 ("Field Width")) -> (s? t:f=w296:u16)
        n205 = property on="Field Width" class="DigNum (strict)"("DisabledEnum"=w299) -> ()  [unwired: 2 in, 2 out]
        n206 = property on="PadType" class="Ring (strict)"("DisabledEnum"=w299) -> ()  [unwired: 2 in, 2 out]
        n207 = property on="Field Width" class="DigNum (strict)"("Value"=w296) -> (error out=w294:errorcluster)  [unwired: 2 in, 1 out]
        n208 = property on="SetFormat" class="Bool (strict)"(error in=w294, "Val(Sgnl)"=TRUE ("Value (Signaling)")) -> ()  [unwired: 1 in, 2 out]
      }
      event "Field Width": Value Change {
        n209 = event-data() -> ("NewVal"=w309:u16)  [unwired: 6 out]
        n210 = property on="SetFormat" class="Bool (strict)"("Val(Sgnl)"=TRUE ("Value (Signaling)")) -> ()  [unwired: 2 in, 2 out]
        n211 = Equal To 0?(x=w309) -> (x = 0?=w305:bool)
        n212 = Select(t=T3."Disabled and Grayed Out" ("Disabled"), s=w305, f=T3."Enabled" ("Disabled")) -> (s? t:f=w306:T3)
        n213 = Select(t=FALSE ("x = 0?"), s=w305, f=TRUE ("x = 0?")) -> (s? t:f=w302:bool)
        n214 = property on="PadType" class="Ring (strict)"("DisabledEnum"=w306) -> ()  [unwired: 2 in, 2 out]
        n215 = property on="Field Width" class="DigNum (strict)"("DisabledEnum"=w306) -> ()  [unwired: 2 in, 2 out]
        n216 = local write "Use minimum field width"(w302) -> ()
      }
      event "TimeFormat": Value Change {
        n217 = event-data() -> ("NewVal"=w314:u16)  [unwired: 6 out]
        n218 = property on="SetFormat" class="Bool (strict)"("Val(Sgnl)"=TRUE ("Value (Signaling)")) -> ()  [unwired: 2 in, 2 out]
        n219 = case shown="0, Default" w314 {
          tunnel: [T3."Enabled" ("Disabled") T3."Disabled and Grayed Out" ("Disabled") T3."Disabled and Grayed Out" ("Disabled")] -> w313
          tunnel: [T3."Enabled" ("Disabled") T3."Enabled" ("Disabled") T3."Disabled and Grayed Out" ("Disabled")] -> w312
          frame 0, Default {
            n220 = property on="HMS" class="Slide (strict)"() -> ("Value"=w315:u16)  [unwired: 2 in, 2 out]
            n221 = property on="HMS" class="Slide (strict)"("Val(Sgnl)"=w315) -> ()  [unwired: 2 in, 2 out]
          }
          frame 1 {
          }
          frame 2 {
          }
        }
        n222 = property on="AMFM" class="Slide (strict)"("DisabledEnum"=w313) -> ()  [unwired: 2 in, 2 out]
        n223 = property on="HMS" class="Slide (strict)"("DisabledEnum"=w313) -> ()  [unwired: 2 in, 2 out]
        n224 = property on="Digits" class="DigNum (strict)"("DisabledEnum"=w312) -> ()  [unwired: 2 in, 2 out]
      }
      event "AMFM", "Digits", "YMD", "YearShow": Value Change {
        n225 = event-data() -> ()  [unwired: 7 out]
        n226 = property on="SetFormat" class="Bool (strict)"("Val(Sgnl)"=TRUE ("Value (Signaling)")) -> ()  [unwired: 2 in, 2 out]
      }
      event "HMS": Value Change {
        n227 = event-data() -> ("NewVal"=w328:u16)  [unwired: 6 out]
        n228 = property on="SetFormat" class="Bool (strict)"("Val(Sgnl)"=TRUE ("Value (Signaling)")) -> ()  [unwired: 2 in, 2 out]
        n229 = Equal To 0?(x=w328) -> (x = 0?=w327:bool)
        n230 = Select(t=T3."Disabled and Grayed Out" ("Disabled"), s=w327, f=T3."Enabled" ("Disabled")) -> (s? t:f=w324:T3)
        n231 = property on="Digits" class="DigNum (strict)"("DisabledEnum"=w324) -> ()  [unwired: 2 in, 2 out]
      }
      event "DateFormat": Value Change {
        n232 = event-data() -> ("NewVal"=w331:u16)  [unwired: 6 out]
        n233 = case shown="1, 2" w331 {
          tunnel: [T3."Enabled" ("Disabled") T3."Disabled and Grayed Out" ("Disabled")] -> w330
          frame 0, Default {
          }
          frame 1, 2 {
          }
        }
        n234 = property on="SetFormat" class="Bool (strict)"("Val(Sgnl)"=TRUE ("Value (Signaling)")) -> ()  [unwired: 2 in, 2 out]
        n235 = property on="YearShow" class="Slide (strict)"("DisabledEnum"=w330) -> ()  [unwired: 2 in, 2 out]
        n236 = property on="YMD" class="Slide (strict)"("DisabledEnum"=w330) -> ()  [unwired: 2 in, 2 out]
      }
      event "Ignore timestamp information": Value Change {
        n237 = event-data() -> ()  [unwired: 7 out]
        n238 = property on="SetFormat" class="Bool (strict)"("Val(Sgnl)"=TRUE ("Value (Signaling)")) -> ()  [unwired: 2 in, 2 out]
      }
      event "SetFormat": Value Change {
        n239 = event-data() -> ()  [unwired: 7 out]
        n240 = local read "Notation"() -> (w335:i32)
        n241 = case shown="0..3, 5..7, Default" w335 {
          tunnel: w335 -> [w348 _]
          tunnel: [w341 w380] -> w336
          frame 0..3, 5..7, Default {
            # "%[$][-][+][#][^][0][Width][.Precision || _SignificantDigits][{Unit}][<Embedded information>]Conversion"
            n242 = local read "Exponent in multiples of 3"() -> (w344:bool)
            n243 = local read "Use minimum field width"() -> (w342:bool)
            n244 = local read "Hide trailing zeros"() -> (w345:bool)
            n245 = local read "PrecisionDigits"() -> (w340:u16)
            n246 = local read "PrecisionType"() -> (w346:u16)
            n247 = local read "Field Width"() -> (w343:u16)
            n248 = local read "PadType"() -> (w347:u16)
            n249 = Select(t="#" ("format string"), s=w345, f="" ("format string")) -> (s? t:f=w357:string)
            n250 = Select(t="^" ("format string"), s=w344, f="" ("format string")) -> (s? t:f=w360:string)
            n251 = case shown="True" w342 {
              tunnel: w347 -> [_ w374]
              tunnel: w343 -> [_ w369]
              tunnel: [w366 w373] -> w362
              tunnel: [w366 w367] -> w363
              tunnel: [w366 w372] -> w361
              frame False {
                w366 = ""
              }
              frame True {
                n252 = Not Equal To 0?(x=w369) -> (x != 0?=w370:bool)
                n253 = case shown="2" w374 {
                  tunnel: [w375 "" ("format string") "0" ("format string")] -> w373
                  tunnel: [w375 "-" ("format string") "" ("format string")] -> w372
                  frame 0, Default {
                    w375 = "" ("format string")
                  }
                  frame 1 {
                  }
                  frame 2 {
                  }
                }
                n254 = Number To Decimal String(number=w369) -> (decimal integer string=w368:string)  [unwired: 1 in]
                n255 = Select(t=w368, s=w370, f="") -> (s? t:f=w367:string)
              }
            }
            n256 = Number To Decimal String(number=w340) -> (decimal integer string=w339:string)  [unwired: 1 in]
            n257 = Equal?(x=w346, y=u16 0) -> (x = y?=w354:bool)
            n258 = Index Array(array=string[] ["f", "e", "g", "p", "", "x", "o", "b", "", "T"], index=w348) -> (element=w365:string)
            n259 = Select(t="." ("format string"), s=w354, f="_" ("format string")) -> (s? t:f=w364:string)
            n260 = Concatenate Strings("%" ("string"), w361, w357, w360, w362, w363, w364, w339, w365) -> (w341:string)
          }
          frame 9 {
            n261 = local read "DateFormat"() -> (w402:u16)
            n262 = local read "TimeFormat"() -> (w398:u16)
            n263 = local read "YearShow"() -> (w404:u16)
            n264 = local read "AMFM"() -> (w399:u16)
            n265 = local read "Digits"() -> (w401:u16)
            n266 = local read "HMS"() -> (w400:u16)
            n267 = local read "YMD"() -> (w403:u16)
            n268 = Equal?(x=w402, y=u16 2) -> (x = y?=w395:bool)
            n269 = Equal?(x=w398, y=u16 2) -> (x = y?=w394:bool)
            n270 = case shown="0, Default" w398 {
              tunnel: w399 -> [w461 _ _]
              tunnel: w400 -> [w459 _ _]
              tunnel: w401 -> [w445 w463 _]
              tunnel: [w448 w462 w465] -> w381
              tunnel: w402 -> [_ _ w470]
              frame 0, Default {
                # "Custom Format"
                n271 = Equal To 0?(x=w461) -> (x = 0?=w452:bool)
                n272 = Not Equal To 0?(x=w445) -> (x != 0?=w447:bool)
                n273 = Equal To 0?(x=w459) -> (x = 0?=w456:bool)
                n274 = Format Into String(format string=":%%S%%%du", w445) -> (resulting string=w444:string)  [unwired: 2 in, 1 out]
                n275 = Select(t="%I:%M" ("format string"), s=w452, f="%H:%M" ("format string")) -> (s? t:f=w457:string)
                n276 = Select(t=w444, s=w447, f=":%S" ("format string")) -> (s? t:f=w443:string)
                n277 = Select(t="", s=w456, f=w443) -> (s? t:f=w453:string)
                n278 = Select(t=" %p", s=w452, f="" ("t")) -> (s? t:f=w449:string)
                n279 = Concatenate Strings(w457, w453, w449) -> (w448:string)
              }
              frame 1 {
                # "System Format"
                n280 = Format Into String(format string="%%.%dX", w463) -> (resulting string=w462:string)  [unwired: 2 in, 1 out]
              }
              frame 2 {
                # "No Used"
                n281 = Equal?(x=w470, y=u16 2) -> (x = y?=w468:bool)
                n282 = Select(t="%.3X" ("format string"), s=w468, f="") -> (s? t:f=w465:string)
              }
            }
            n283 = case shown="0, Default" w402 {
              tunnel: w403 -> [w411 _ _]
              tunnel: w404 -> [w410 _ _]
              tunnel: [w408 "%x" ("format string") w437] -> w382
              tunnel: w398 -> [_ _ w438]
              frame 0, Default {
                # "Custom Format"
                n284 = case shown="2" w410 {
                  tunnel: ["" ("format string") "%y" ("format string") "%Y" ("format string")] -> w409
                  frame 0, Default {
                  }
                  frame 1 {
                  }
                  frame 2 {
                  }
                }
                n285 = case shown="2" w411 {
                  tunnel: w409 -> [w416 w423 w431]
                  tunnel: [w420 w427 w435] -> w408
                  frame 0, Default {
                    n286 = Empty String/Path?(string/path=w416) -> (empty?=w419:bool)
                    n287 = Concatenate Strings("/" ("string"), w416) -> (w417:string)
                    n288 = Select(t=w416, s=w419, f=w417) -> (s? t:f=w418:string)
                    n289 = Concatenate Strings("%m/%d" ("format string"), w418) -> (w420:string)
                  }
                  frame 1 {
                    n290 = Empty String/Path?(string/path=w423) -> (empty?=w426:bool)
                    n291 = Concatenate Strings("/" ("string"), w423) -> (w424:string)
                    n292 = Select(t=w423, s=w426, f=w424) -> (s? t:f=w425:string)
                    n293 = Concatenate Strings("%d/%m" ("format string"), w425) -> (w427:string)
                  }
                  frame 2 {
                    n294 = Empty String/Path?(string/path=w431) -> (empty?=w434:bool)
                    n295 = Concatenate Strings(w431, "/" ("string")) -> (w433:string)
                    n296 = Select(t=w431, s=w434, f=w433) -> (s? t:f=w430:string)
                    n297 = Concatenate Strings(w430, "%m/%d" ("format string")) -> (w435:string)
                  }
                }
              }
              frame 1 {
                # "System Format"
              }
              frame 2 {
                # "No Used"
                n298 = Equal?(x=w438, y=u16 2) -> (x = y?=w440:bool)
                n299 = Select(t="%x" ("format string"), s=w440, f="") -> (s? t:f=w437:string)
              }
            }
            n300 = Compound Arithmetic op=AND(w395, w394) -> (w387:bool)
            n301 = Compound Arithmetic op=AND(invert w395, w394) -> (w391:bool)
            n302 = Compound Arithmetic op=AND(w395, invert w394) -> (w392:bool)
            n303 = Compound Arithmetic op=AND(invert w395, invert w394) -> (w396:bool)
            n304 = Compound Arithmetic op=OR(w391, w392) -> (w393:bool)
            n305 = Build Array(w387, w393, w396) -> (w388:bool[])
            n306 = Search 1D Array(1D array=w388, element=TRUE) -> (index of element=w390:i32)  [unwired: 1 in]
            n307 = case shown="2" w390 {
              tunnel: [" " ("format string") "" ("format string") "\n" ("format string")] -> w397
              frame 0, Default {
              }
              frame 1 {
              }
              frame 2 {
              }
            }
            n308 = Concatenate Strings("%<" ("string"), w381, w397, w382, ">T" ("string")) -> (w380:string)
          }
        }
        n309 = local read "FormatAxis"() -> (w338:u16)
        n310 = case shown="0, Default" w338 {
          tunnel: w337 -> [w472 w475 w478]
          tunnel: w336 -> [w471 w473 w476]
          frame 0, Default {
            n311 = property class="WFGraph"(reference=w472, "XScale.FormatString"=w471) -> ()  [unwired: 1 in, 2 out]
          }
          frame 1 {
            n312 = property class="WFGraph"(reference=w475, "ActYScl"=0 ("Active Y Scale"), "YScale.FormatString"=w473) -> ()  [unwired: 1 in, 2 out]
          }
          frame 2 {
            n313 = property class="WFGraph"(reference=w478, "ActYScl"=1 ("Active Y Scale"), "YScale.FormatString"=w476) -> ()  [unwired: 1 in, 2 out]
          }
        }
      }
      event "LineStyle0", "LineStyle1", "LineStyle2", "LineStyle3", "LineStyle4": Value Change {
        n314 = event-data() -> ("CtlRef"=w485:refnum<vi>)  [unwired: 6 out]
        n315 = property class="Bool (strict)"(reference=w485) -> ("Label.Text"=w483:string)  [unwired: 1 in, 2 out]
        n316 = local read "LineStyle"() -> (w482:string)
        n317 = Equal?(x=w483, y=w482) -> (x = y?=w484:bool)
        n318 = case shown="False" w484 {
          tunnel: w483 -> [w494 w507]
          tunnel: w482 -> [w500 _]
          tunnel: w481 -> [w490 _]
          tunnel: w480 -> [w488 _]
          tunnel: w479 -> [w487 _]
          frame False {
            n319 = control-ref of="This VI"() -> (w501:refnum<vi>)
            n320 = Match Pattern(string=w494, regular expression="LineStyle") -> (after substring=w492:string)  [unwired: 4 out]
            n321 = To Variant(anything=TRUE) -> (Variant=w498:variant)
            n322 = Decimal String To Number(string=w492) -> (number=w491:i32)  [unwired: 3 out]
            n323 = invoke class="VI" method="Ctrl Val.Set"(reference=w501, "Control Name"=w494, "Value"=w498) -> (reference out=w499:refnum<vi>)  [unwired: 2 in, 4 out]
            n324 = To Unsigned Byte Integer(number=w491) -> (unsigned 8bit integer=w486:u8)
            n325 = local write "LineStyle"(w494) -> ()
            n326 = To Variant(anything=FALSE) -> (Variant=w496:variant)
            n327 = property class="WFGraph"(reference=w490, "Plot.Line Style"=w486) -> ()  [unwired: 1 in, 2 out]
            n328 = invoke class="VI" method="Ctrl Val.Set"(reference=w499, "Control Name"=w500, "Value"=w496) -> ()  [unwired: 2 in, 5 out]
            n329 = property on="Items" class="Ring (strict)"() -> ("Value"=w489:u16)  [unwired: 2 in, 2 out]
            n330 = case shown="Default" w488 {
              tunnel: w487 -> [_ w505]
              tunnel: w486 -> [_ w502]
              tunnel: w489 -> [_ w504]
              frame "ViewReport" {
              }
              frame Default {
                n331 = call "CRYSet Plot Settings.vi"("Style"=w502, "sAction"="LineStyle", "Row"=w504, "Legend Refnum"=w505, "Type"=enum16{"Curves", "Values", "Results", "WFM"}."WFM") -> ()  [unwired: 2 in, 5 out]
              }
            }
          }
          frame True {
            n332 = control-ref of="This VI"() -> (w510:refnum<vi>)
            n333 = To Variant(anything=TRUE) -> (Variant=w509:variant)
            n334 = invoke class="VI" method="Ctrl Val.Set"(reference=w510, "Control Name"=w507, "Value"=w509) -> ()  [unwired: 2 in, 5 out]
          }
        }
      }
      event "LineWidth0", "LineWidth1", "LineWidth2", "LineWidth3", "LineWidth4", "LineWidth5": Value Change {
        n335 = event-data() -> ("CtlRef"=w514:refnum<vi>)  [unwired: 6 out]
        n336 = property class="Bool (strict)"(reference=w514) -> ("Label.Text"=w516:string)  [unwired: 1 in, 2 out]
        n337 = local read "LineWidth"() -> (w515:string)
        n338 = Equal?(x=w516, y=w515) -> (x = y?=w517:bool)
        n339 = case shown="False" w517 {
          tunnel: w516 -> [w524 w539]
          tunnel: w515 -> [w532 _]
          tunnel: w513 -> [w522 _]
          tunnel: w512 -> [w520 _]
          tunnel: w511 -> [w519 _]
          frame False {
            n340 = control-ref of="This VI"() -> (w533:refnum<vi>)
            n341 = Match Pattern(string=w524, regular expression="LineWidth") -> (after substring=w525:string)  [unwired: 4 out]
            n342 = To Variant(anything=TRUE) -> (Variant=w530:variant)
            n343 = Decimal String To Number(string=w525) -> (number=w526:i32)  [unwired: 3 out]
            n344 = invoke class="VI" method="Ctrl Val.Set"(reference=w533, "Control Name"=w524, "Value"=w530) -> (reference out=w531:refnum<vi>)  [unwired: 2 in, 4 out]
            n345 = To Unsigned Byte Integer(number=w526) -> (unsigned 8bit integer=w518:u8)
            n346 = local write "LineWidth"(w524) -> ()
            n347 = To Variant(anything=FALSE) -> (Variant=w528:variant)
            n348 = property class="WFGraph"(reference=w522, "Plot.Line Width"=w518) -> ()  [unwired: 1 in, 2 out]
            n349 = invoke class="VI" method="Ctrl Val.Set"(reference=w531, "Control Name"=w532, "Value"=w528) -> ()  [unwired: 2 in, 5 out]
            n350 = property on="Items" class="Ring (strict)"() -> ("Value"=w521:u16)  [unwired: 2 in, 2 out]
            n351 = case shown="Default" w520 {
              tunnel: w519 -> [_ w537]
              tunnel: w518 -> [_ w534]
              tunnel: w521 -> [_ w536]
              frame "ViewReport" {
              }
              frame Default {
                n352 = call "CRYSet Plot Settings.vi"("Style"=w534, "sAction"="LineWidth", "Row"=w536, "Legend Refnum"=w537, "Type"=enum16{"Curves", "Values", "Results", "WFM"}."WFM") -> ()  [unwired: 2 in, 5 out]
              }
            }
          }
          frame True {
            n353 = control-ref of="This VI"() -> (w542:refnum<vi>)
            n354 = To Variant(anything=TRUE) -> (Variant=w541:variant)
            n355 = invoke class="VI" method="Ctrl Val.Set"(reference=w542, "Control Name"=w539, "Value"=w541) -> ()  [unwired: 2 in, 5 out]
          }
        }
      }
      event "PointStyle0", "PointStyle1", "PointStyle2", "PointStyle3", "PointStyle4", "PointStyle5", "PointStyle6", "PointStyle7", "PointStyle8", "PointStyle9", "PointStyle10", "PointStyle11", "PointStyle12", "PointStyle13", "PointStyle14", "PointStyle15", "PointStyle16": Value Change {
        n356 = event-data() -> ("CtlRef"=w546:refnum<vi>)  [unwired: 6 out]
        n357 = property class="Bool (strict)"(reference=w546) -> ("Label.Text"=w548:string)  [unwired: 1 in, 2 out]
        n358 = local read "PointStyle"() -> (w547:string)
        n359 = Equal?(x=w548, y=w547) -> (x = y?=w549:bool)
        n360 = case shown="False" w549 {
          tunnel: w548 -> [w556 w571]
          tunnel: w547 -> [w564 _]
          tunnel: w545 -> [w554 _]
          tunnel: w544 -> [w552 _]
          tunnel: w543 -> [w551 _]
          frame False {
            n361 = control-ref of="This VI"() -> (w565:refnum<vi>)
            n362 = To Variant(anything=TRUE) -> (Variant=w562:variant)
            n363 = Match Pattern(string=w556, regular expression="PointStyle") -> (after substring=w557:string)  [unwired: 4 out]
            n364 = invoke class="VI" method="Ctrl Val.Set"(reference=w565, "Control Name"=w556, "Value"=w562) -> (reference out=w563:refnum<vi>)  [unwired: 2 in, 4 out]
            n365 = Decimal String To Number(string=w557) -> (number=w558:i32)  [unwired: 3 out]
            n366 = local write "PointStyle"(w556) -> ()
            n367 = To Variant(anything=FALSE) -> (Variant=w560:variant)
            n368 = To Unsigned Byte Integer(number=w558) -> (unsigned 8bit integer=w550:u8)
            n369 = invoke class="VI" method="Ctrl Val.Set"(reference=w563, "Control Name"=w564, "Value"=w560) -> ()  [unwired: 2 in, 5 out]
            n370 = property class="WFGraph"(reference=w554, "Plot.Point Style"=w550) -> ()  [unwired: 1 in, 2 out]
            n371 = property on="Items" class="Ring (strict)"() -> ("Value"=w553:u16)  [unwired: 2 in, 2 out]
            n372 = case shown="Default" w552 {
              tunnel: w551 -> [_ w569]
              tunnel: w550 -> [_ w566]
              tunnel: w553 -> [_ w568]
              frame "ViewReport" {
              }
              frame Default {
                n373 = call "CRYSet Plot Settings.vi"("Style"=w566, "sAction"="PointStyle", "Row"=w568, "Legend Refnum"=w569, "Type"=enum16{"Curves", "Values", "Results", "WFM"}."WFM") -> ()  [unwired: 2 in, 5 out]
              }
            }
          }
          frame True {
            n374 = control-ref of="This VI"() -> (w574:refnum<vi>)
            n375 = To Variant(anything=TRUE) -> (Variant=w573:variant)
            n376 = invoke class="VI" method="Ctrl Val.Set"(reference=w574, "Control Name"=w571, "Value"=w573) -> ()  [unwired: 2 in, 5 out]
          }
        }
      }
      event "Interpolation0", "Interpolation1", "Interpolation2", "Interpolation3", "Interpolation4", "Interpolation5": Value Change {
        n377 = event-data() -> ("CtlRef"=w578:refnum<vi>)  [unwired: 6 out]
        n378 = property class="Bool (strict)"(reference=w578) -> ("Label.Text"=w580:string)  [unwired: 1 in, 2 out]
        n379 = local read "Interpolation"() -> (w579:string)
        n380 = Equal?(x=w580, y=w579) -> (x = y?=w581:bool)
        n381 = case shown="False" w581 {
          tunnel: w580 -> [w588 w603]
          tunnel: w579 -> [w596 _]
          tunnel: w577 -> [w586 _]
          tunnel: w576 -> [w584 _]
          tunnel: w575 -> [w583 _]
          frame False {
            n382 = control-ref of="This VI"() -> (w597:refnum<vi>)
            n383 = To Variant(anything=TRUE) -> (Variant=w594:variant)
            n384 = Match Pattern(string=w588, regular expression="Interpolation") -> (after substring=w589:string)  [unwired: 4 out]
            n385 = invoke class="VI" method="Ctrl Val.Set"(reference=w597, "Control Name"=w588, "Value"=w594) -> (reference out=w595:refnum<vi>)  [unwired: 2 in, 4 out]
            n386 = Decimal String To Number(string=w589) -> (number=w590:i32)  [unwired: 3 out]
            n387 = local write "Interpolation"(w588) -> ()
            n388 = To Variant(anything=FALSE) -> (Variant=w592:variant)
            n389 = To Unsigned Byte Integer(number=w590) -> (unsigned 8bit integer=w582:u8)
            n390 = invoke class="VI" method="Ctrl Val.Set"(reference=w595, "Control Name"=w596, "Value"=w592) -> ()  [unwired: 2 in, 5 out]
            n391 = property class="WFGraph"(reference=w586, "Plot.Plot Interpolation"=w582) -> ()  [unwired: 1 in, 2 out]
            n392 = property on="Items" class="Ring (strict)"() -> ("Value"=w585:u16)  [unwired: 2 in, 2 out]
            n393 = case shown="Default" w584 {
              tunnel: w583 -> [_ w601]
              tunnel: w582 -> [_ w598]
              tunnel: w585 -> [_ w600]
              frame "ViewReport" {
              }
              frame Default {
                n394 = call "CRYSet Plot Settings.vi"("Style"=w598, "sAction"="Interpolation", "Row"=w600, "Legend Refnum"=w601, "Type"=enum16{"Curves", "Values", "Results", "WFM"}."WFM") -> ()  [unwired: 2 in, 5 out]
              }
            }
          }
          frame True {
            n395 = control-ref of="This VI"() -> (w606:refnum<vi>)
            n396 = To Variant(anything=TRUE) -> (Variant=w605:variant)
            n397 = invoke class="VI" method="Ctrl Val.Set"(reference=w606, "Control Name"=w603, "Value"=w605) -> ()  [unwired: 2 in, 5 out]
          }
        }
      }
      event "Items": Value Change {
        n398 = event-data() -> ("NewVal"=w608:u16)  [unwired: 6 out]
        n399 = flat-sequence {
          tunnel: w607 -> [w614]
          tunnel: w608 -> [w613]
          tunnel: w609 -> [w611]
          tunnel: [w623] -> w610
          tunnel: w610 -> [w636]
          tunnel: w608 -> [w635]
          tunnel: w607 -> [w633]
          frame #0 {
            n400 = property class="MCListbox"(reference=w611) -> ("ItemSyms"=w615:i32[])  [unwired: 1 in, 2 out]
            n401 = Index Array(array=w615, index=w613) -> (element=w617:i32)
            n402 = Equal?(x=w617, y=38) -> (x = y?=w612:bool)
            n403 = property class="WFGraph"(reference=w614, "Active Plot"=w613, "Plot.Visible?"=w612) -> ()  [unwired: 1 in, 2 out]
            n404 = local write "Show Plot"(w612) -> ()
          }
          frame #1 {
            n405 = local read "Interpolation"() -> (w619:string)
            n406 = local read "LineWidth"() -> (w621:string)
            n407 = local read "PointStyle"() -> (w620:string)
            n408 = local read "LineStyle"() -> (w622:string)
            n409 = control-ref of="This VI"() -> (w623:refnum<vi>)
            n410 = To Variant(anything=FALSE) -> (Variant=w624:variant)
            n411 = invoke class="VI" method="Ctrl Val.Set"(reference=w623, "Control Name"=w622, "Value"=w624) -> ()  [unwired: 2 in, 5 out]
            n412 = invoke class="VI" method="Ctrl Val.Set"(reference=w623, "Control Name"=w621, "Value"=w624) -> ()  [unwired: 2 in, 5 out]
            n413 = invoke class="VI" method="Ctrl Val.Set"(reference=w623, "Control Name"=w620, "Value"=w624) -> ()  [unwired: 2 in, 5 out]
            n414 = invoke class="VI" method="Ctrl Val.Set"(reference=w623, "Control Name"=w619, "Value"=w624) -> ()  [unwired: 2 in, 5 out]
          }
          frame #2 {
            n415 = call "CRYGet Line Infor.vi"("This VI"=w636, "Active Plot Number"=w635, "Graph Type"="WAVE", "Wave Graph Control Ref"=w633, "Property Set?"=TRUE) -> ("Line"=w625:u32, "Point/Fill"=w626:u32, "Fill to"=w627:i16, "LineStyle"=w632:string, "LineWidth"=w631:string, "PointStyle"=w630:string, "Interpolation"=w629:string)  [unwired: 16 in]
            n416 = local write "Interpolation"(w629) -> ()
            n417 = local write "LineWidth"(w631) -> ()
            n418 = local write "Point/Fill"(w626) -> ()
            n419 = local write "LineStyle"(w632) -> ()
            n420 = local write "PointStyle"(w630) -> ()
            n421 = local write "Fill to"(w627) -> ()
            n422 = local write "Line"(w625) -> ()
          }
        }
      }
      event "Show Plot": Value Change {
        w644 = 38
        n423 = event-data() -> ("NewVal"=w637:bool)  [unwired: 6 out]
        n424 = local read "Items"() -> (w638:u16)
        n425 = property class="MCListbox"(reference=w639) -> (reference out=w642:refnum<vi>, "ItemSyms"=w647:i32[])  [unwired: 1 in, 1 out]
        n426 = property class="WFGraph"(reference=w640, "Active Plot"=w638, "Plot.Visible?"=w637) -> ()  [unwired: 1 in, 2 out]
        n427 = Index Array(array=w647, index=w638) -> (element=w641:i32)
        n428 = Equal?(x=w641, y=w644) -> (x = y?=w643:bool)
        n429 = Select(t=37, s=w643, f=w644) -> (s? t:f=w646:i32)
        n430 = Replace Array Subset(array=w647, new element=w646, index=w638) -> (w648:i32[])
        n431 = property class="MCListbox"(reference=w642, "ItemSyms"=w648) -> ()  [unwired: 1 in, 2 out]
      }
      event "Line": Value Change {
        n432 = event-data() -> ("NewVal"=w652:u32)  [unwired: 6 out]
        n433 = property class="WFGraph"(reference=w656, "Plot.Plot Color"=w652) -> ()  [unwired: 1 in, 2 out]
        n434 = property on="Items" class="Ring (strict)"() -> ("Value"=w649:u16)  [unwired: 2 in, 2 out]
        n435 = Bundle By Name(cluster=T4 {"Row"=0, "Column"=0} ("Active Cell:Active Cell"), "Row"=w649, "Column"=1) -> (w653:T4)
        n436 = case shown="Default" w650 {
          tunnel: w655 -> [_ w660]
          tunnel: w652 -> [_ w659]
          tunnel: w649 -> [_ w658]
          frame "ViewReport" {
          }
          frame Default {
            n437 = call "CRYSet Plot Settings.vi"("sAction"="Color", "Color"=w659, "Row"=w658, "Legend Refnum"=w660, "Type"=enum16{"Curves", "Values", "Results", "WFM"}."WFM") -> ()  [unwired: 2 in, 5 out]
          }
        }
        n438 = property class="MCListbox"(reference=w655, "ActiveCell"=w653, "CellBG"=w652) -> ()  [unwired: 1 in, 2 out]
      }
      event "Point/Fill": Value Change {
        n439 = event-data() -> ("NewVal"=w662:u32)  [unwired: 6 out]
        n440 = property class="WFGraph"(reference=w666, "Plot.Fill/Pt. Color"=w662) -> ()  [unwired: 1 in, 2 out]
        n441 = property on="Items" class="Ring (strict)"() -> ("Value"=w665:u16)  [unwired: 2 in, 2 out]
        n442 = case shown="Default" w664 {
          tunnel: w663 -> [_ w670]
          tunnel: w662 -> [_ w669]
          tunnel: w665 -> [_ w668]
          frame "ViewReport" {
          }
          frame Default {
            n443 = call "CRYSet Plot Settings.vi"("sAction"="PointColor", "Color"=w669, "Row"=w668, "Legend Refnum"=w670, "Type"=enum16{"Curves", "Values", "Results", "WFM"}."WFM") -> ()  [unwired: 2 in, 5 out]
          }
        }
      }
      event "Fill to": Value Change {
        n444 = event-data() -> ("NewVal"=w672:i16)  [unwired: 6 out]
        n445 = property class="WFGraph"(reference=w676, "Plot.Fill To"=w672) -> ()  [unwired: 1 in, 2 out]
        n446 = property on="Items" class="Ring (strict)"() -> ("Value"=w675:u16)  [unwired: 2 in, 2 out]
        n447 = case shown="Default" w673 {
          tunnel: w674 -> [_ w680]
          tunnel: w672 -> [_ w677]
          tunnel: w675 -> [_ w679]
          frame "ViewReport" {
          }
          frame Default {
            n448 = call "CRYSet Plot Settings.vi"("Fill To"=w677, "sAction"="FillTo", "Row"=w679, "Legend Refnum"=w680, "Type"=enum16{"Curves", "Values", "Results", "WFM"}."WFM") -> ()  [unwired: 2 in, 5 out]
          }
        }
      }
      event "ScaleAxis": Value Change {
        n449 = event-data() -> ("NewVal"=w703:u16)  [unwired: 6 out]
        n450 = case shown="0, Default" w703 {
          tunnel: w704 -> [w717 w731 w745]
          tunnel: [w716 w730 w744] -> w698
          tunnel: [w715 w729 w743] -> w692
          tunnel: [w714 w728 w742] -> w694
          tunnel: [w713 w727 w741] -> w691
          tunnel: [w712 w726 w740] -> w689
          tunnel: [w711 w725 w739] -> w688
          tunnel: [w710 w724 w738] -> w687
          tunnel: [w709 w723 w737] -> w686
          tunnel: [w708 w722 w736] -> w685
          tunnel: [w707 w721 w735] -> w684
          tunnel: [w706 w720 w734] -> w683
          tunnel: [w705 w718 w732] -> w682
          frame 0, Default {
            n451 = property class="WFGraph"(reference=w717) -> ("XScale.NameLbl.Visible"=w716:bool, "XScale.Style"=w715:u8, "XScale.Mapping Mode"=w714:u8, "XScale.ScaleFit"=w713:u8, "XScale.Maximum"=w712:dbl, "XScale.Minimum"=w711:dbl, "XScale.TickColor"=w710:u32, "XScale.MinorTickColor"=w709:u32, "XScale.Text Color"=w708:u32, "XScale.MajGrdColor"=w707:u32, "XScale.MnrGrdColor"=w706:u32, "XScale.NameLbl.Text"=w705:string)  [unwired: 1 in, 2 out]
          }
          frame 1 {
            n452 = property class="WFGraph"(reference=w731, "ActXScl"=0 ("Active X Scale")) -> ("YScale.NameLbl.Visible"=w730:bool, "YScale.Style"=w729:u8, "YScale.Mapping Mode"=w728:u8, "YScale.ScaleFit"=w727:u8, "YScale.Maximum"=w726:dbl, "YScale.Minimum"=w725:dbl, "YScale.TickColor"=w724:u32, "YScale.MinorTickColor"=w723:u32, "YScale.Text Color"=w722:u32, "YScale.MajGrdColor"=w721:u32, "YScale.MnrGrdColor"=w720:u32, "YScale.NameLbl.Text"=w718:string)  [unwired: 1 in, 2 out]
          }
          frame 2 {
            n453 = property class="WFGraph"(reference=w745, "ActXScl"=1 ("Active X Scale")) -> ("YScale.NameLbl.Visible"=w744:bool, "YScale.Style"=w743:u8, "YScale.Mapping Mode"=w742:u8, "YScale.ScaleFit"=w741:u8, "YScale.Maximum"=w740:dbl, "YScale.Minimum"=w739:dbl, "YScale.TickColor"=w738:u32, "YScale.MinorTickColor"=w737:u32, "YScale.Text Color"=w736:u32, "YScale.MajGrdColor"=w735:u32, "YScale.MnrGrdColor"=w734:u32, "YScale.NameLbl.Text"=w732:string)  [unwired: 1 in, 2 out]
          }
        }
        n454 = Equal?(x=w694, y=u8 1 ("X Scale.Scale Fit")) -> (x = y?=w693:bool)
        n455 = Not Equal?(x=w692, y=u8 5 ("X Scale.Scale Fit")) -> (x != y?=w696:bool)
        n456 = Equal?(x=w691, y=u8 2 ("X Scale.Scale Fit")) -> (x = y?=w690:bool)
        n457 = local write "Show scale label"(w698) -> ()
        n458 = local write "Show scale"(w696) -> ()
        n459 = local write "Scale Style"(w692) -> ()
        n460 = local write "Log"(w693) -> ()
        n461 = local write "Minor grid"(w683) -> ()
        n462 = local write "Minimum"(w688) -> ()
        n463 = local write "Minor tick"(w686) -> ()
        n464 = local write "Major grid"(w684) -> ()
        n465 = local write "Autoscale"(w690) -> ()
        n466 = local write "Maximum"(w689) -> ()
        n467 = local write "Major tick"(w687) -> ()
        n468 = local write "Marker text"(w685) -> ()
        n469 = local write "Axis Name"(w682) -> ()
        n470 = Select(t=u8 2 ("X Scale.Scale Fit"), s=w690, f=u8 0 ("X Scale.Scale Fit")) -> (s? t:f=w702:u8)
        n471 = property on="Maximum" class="DigNum (strict)"("Disabled"=w702) -> ()  [unwired: 2 in, 2 out]
        n472 = property on="Minimum" class="DigNum (strict)"("Disabled"=w702) -> ()  [unwired: 2 in, 2 out]
      }
      event "Axis Name": Value Change {
        n473 = event-data() -> ("NewVal"=w748:string)  [unwired: 6 out]
        n474 = local read "ScaleAxis"() -> (w747:u16)
        n475 = local write "Axis Name"(w748) -> ()
        n476 = case shown="0, Default" w747 {
          tunnel: w746 -> [w750 w753 w756]
          tunnel: w748 -> [w749 w751 w754]
          frame 0, Default {
            n477 = property class="WFGraph"(reference=w750, "XScale.NameLbl.Text"=w749) -> ()  [unwired: 1 in, 2 out]
          }
          frame 1 {
            n478 = property class="WFGraph"(reference=w753, "ActYScl"=0 ("Active Y Scale"), "YScale.NameLbl.Text"=w751) -> ()  [unwired: 1 in, 2 out]
          }
          frame 2 {
            n479 = property class="WFGraph"(reference=w756, "ActYScl"=1 ("Active Y Scale"), "YScale.NameLbl.Text"=w754) -> ()  [unwired: 1 in, 2 out]
          }
        }
      }
      event "Show scale label": Value Change {
        n480 = event-data() -> ("NewVal"=w758:bool)  [unwired: 6 out]
        n481 = local read "ScaleAxis"() -> (w759:u16)
        n482 = case shown="0, Default" w759 {
          tunnel: w757 -> [w761 w764 w767]
          tunnel: w758 -> [w760 w762 w765]
          frame 0, Default {
            n483 = property class="WFGraph"(reference=w761, "XScale.NameLbl.Visible"=w760) -> ()  [unwired: 1 in, 2 out]
          }
          frame 1 {
            n484 = property class="WFGraph"(reference=w764, "ActYScl"=0 ("Active Y Scale"), "YScale.NameLbl.Visible"=w762) -> ()  [unwired: 1 in, 2 out]
          }
          frame 2 {
            n485 = property class="WFGraph"(reference=w767, "ActYScl"=1 ("Active Y Scale"), "YScale.NameLbl.Visible"=w765) -> ()  [unwired: 1 in, 2 out]
          }
        }
      }
      event "Show scale": Value Change {
        n486 = event-data() -> ("NewVal"=w768:bool)  [unwired: 6 out]
        n487 = local read "Scale Style"() -> (w772:u8)
        n488 = Equal?(x=u8 5 ("X Scale.Scale Fit"), y=w772) -> (x = y?=w775:bool)
        n489 = Select(t=u8 0 ("X Scale.Scale Fit"), s=w775, f=w772) -> (s? t:f=w777:u8)
        n490 = Select(t=w777, s=w768, f=u8 5 ("X Scale.Scale Fit")) -> (s? t:f=w771:u8)
        n491 = local read "ScaleAxis"() -> (w769:u16)
        n492 = local write "Scale Style"(w771) -> ()
        n493 = case shown="0, Default" w769 {
          tunnel: w771 -> [w779 w781 w783]
          tunnel: w770 -> [w778 w782 w785]
          frame 0, Default {
            n494 = property class="WFGraph"(reference=w778, "XScale.Style"=w779) -> ()  [unwired: 1 in, 2 out]
          }
          frame 1 {
            n495 = property class="WFGraph"(reference=w782, "ActYScl"=0 ("Active Y Scale"), "YScale.Style"=w781) -> ()  [unwired: 1 in, 2 out]
          }
          frame 2 {
            n496 = property class="WFGraph"(reference=w785, "ActYScl"=1 ("Active Y Scale"), "YScale.Style"=w783) -> ()  [unwired: 1 in, 2 out]
          }
        }
      }
      event "Log": Value Change {
        n497 = event-data() -> ("NewVal"=w788:bool)  [unwired: 6 out]
        n498 = Select(t=u8 1 ("X Scale.Scale Fit"), s=w788, f=u8 0 ("X Scale.Scale Fit")) -> (s? t:f=w791:u8)
        n499 = local read "ScaleAxis"() -> (w787:u16)
        n500 = case shown="2" w787 {
          tunnel: w791 -> [w793 w795 w797]
          tunnel: w786 -> [w792 w796 w799]
          frame 0, Default {
            n501 = property class="WFGraph"(reference=w792, "XScale.Mapping Mode"=w793) -> ()  [unwired: 1 in, 2 out]
          }
          frame 1 {
            n502 = property class="WFGraph"(reference=w796, "ActYScl"=0 ("Active Y Scale"), "YScale.Mapping Mode"=w795) -> ()  [unwired: 1 in, 2 out]
          }
          frame 2 {
            n503 = property class="WFGraph"(reference=w799, "ActYScl"=1 ("Active Y Scale"), "YScale.Mapping Mode"=w797) -> ()  [unwired: 1 in, 2 out]
          }
        }
      }
      event "GridStyle": Value Change {
        n504 = event-data() -> ("NewVal"=w801:u16)  [unwired: 6 out]
        n505 = local read "ScaleAxis"() -> (w802:u16)
        n506 = case shown="2" w802 {
          tunnel: w801 -> [w804 w806 w808]
          tunnel: w800 -> [w803 w807 w810]
          frame 0, Default {
            n507 = property class="WFGraph"(reference=w803, "XScale.Style"=w804) -> ()  [unwired: 1 in, 2 out]
          }
          frame 1 {
            n508 = property class="WFGraph"(reference=w807, "ActYScl"=0 ("Active Y Scale"), "YScale.Style"=w806) -> ()  [unwired: 1 in, 2 out]
          }
          frame 2 {
            n509 = property class="WFGraph"(reference=w810, "ActYScl"=1 ("Active Y Scale"), "YScale.Style"=w808) -> ()  [unwired: 1 in, 2 out]
          }
        }
      }
      event "Major tick": Value Change {
        n510 = event-data() -> ("NewVal"=w812:u32)  [unwired: 6 out]
        n511 = local read "ScaleAxis"() -> (w813:u16)
        n512 = case shown="0, Default" w813 {
          tunnel: w811 -> [w815 w818 w821]
          tunnel: w812 -> [w814 w816 w819]
          frame 0, Default {
            n513 = property class="WFGraph"(reference=w815, "XScale.TickColor"=w814) -> ()  [unwired: 1 in, 2 out]
          }
          frame 1 {
            n514 = property class="WFGraph"(reference=w818, "ActYScl"=0 ("Active Y Scale"), "YScale.TickColor"=w816) -> ()  [unwired: 1 in, 2 out]
          }
          frame 2 {
            n515 = property class="WFGraph"(reference=w821, "ActYScl"=1 ("Active Y Scale"), "YScale.TickColor"=w819) -> ()  [unwired: 1 in, 2 out]
          }
        }
      }
      event "Minor tick": Value Change {
        n516 = event-data() -> ("NewVal"=w823:u32)  [unwired: 6 out]
        n517 = local read "ScaleAxis"() -> (w824:u16)
        n518 = case shown="0, Default" w824 {
          tunnel: w823 -> [w826 w828 w830]
          tunnel: w822 -> [w825 w829 w832]
          frame 0, Default {
            n519 = property class="WFGraph"(reference=w825, "XScale.MinorTickColor"=w826) -> ()  [unwired: 1 in, 2 out]
          }
          frame 1 {
            n520 = property class="WFGraph"(reference=w829, "ActYScl"=0 ("Active Y Scale"), "YScale.MinorTickColor"=w828) -> ()  [unwired: 1 in, 2 out]
          }
          frame 2 {
            n521 = property class="WFGraph"(reference=w832, "ActYScl"=1 ("Active Y Scale"), "YScale.MinorTickColor"=w830) -> ()  [unwired: 1 in, 2 out]
          }
        }
      }
      event "Marker text": Value Change {
        n522 = event-data() -> ("NewVal"=w834:u32)  [unwired: 6 out]
        n523 = local read "ScaleAxis"() -> (w835:u16)
        n524 = case shown="0, Default" w835 {
          tunnel: w834 -> [w837 w839 w841]
          tunnel: w833 -> [w836 w840 w843]
          frame 0, Default {
            n525 = property class="WFGraph"(reference=w836, "XScale.Text Color"=w837) -> ()  [unwired: 1 in, 2 out]
          }
          frame 1 {
            n526 = property class="WFGraph"(reference=w840, "ActYScl"=0 ("Active Y Scale"), "YScale.Text Color"=w839) -> ()  [unwired: 1 in, 2 out]
          }
          frame 2 {
            n527 = property class="WFGraph"(reference=w843, "ActYScl"=1 ("Active Y Scale"), "YScale.Text Color"=w841) -> ()  [unwired: 1 in, 2 out]
          }
        }
      }
      event "Major grid": Value Change {
        n528 = event-data() -> ("NewVal"=w846:u32)  [unwired: 6 out]
        n529 = local read "ScaleAxis"() -> (w845:u16)
        n530 = case shown="0, Default" w845 {
          tunnel: w846 -> [w848 w850 w852]
          tunnel: w844 -> [w847 w851 w854]
          frame 0, Default {
            n531 = property class="WFGraph"(reference=w847, "XScale.MajGrdColor"=w848) -> ()  [unwired: 1 in, 2 out]
          }
          frame 1 {
            n532 = property class="WFGraph"(reference=w851, "ActYScl"=0 ("Active Y Scale"), "YScale.MajGrdColor"=w850) -> ()  [unwired: 1 in, 2 out]
          }
          frame 2 {
            n533 = property class="WFGraph"(reference=w854, "ActYScl"=1 ("Active Y Scale"), "YScale.MajGrdColor"=w852) -> ()  [unwired: 1 in, 2 out]
          }
        }
      }
      event "Minor grid": Value Change {
        n534 = event-data() -> ("NewVal"=w856:u32)  [unwired: 6 out]
        n535 = local read "ScaleAxis"() -> (w857:u16)
        n536 = case shown="0, Default" w857 {
          tunnel: w856 -> [w859 w861 w863]
          tunnel: w855 -> [w858 w862 w865]
          frame 0, Default {
            n537 = property class="WFGraph"(reference=w858, "XScale.MnrGrdColor"=w859) -> ()  [unwired: 1 in, 2 out]
          }
          frame 1 {
            n538 = property class="WFGraph"(reference=w862, "ActYScl"=0 ("Active Y Scale"), "YScale.MnrGrdColor"=w861) -> ()  [unwired: 1 in, 2 out]
          }
          frame 2 {
            n539 = property class="WFGraph"(reference=w865, "ActYScl"=1 ("Active Y Scale"), "YScale.MnrGrdColor"=w863) -> ()  [unwired: 1 in, 2 out]
          }
        }
      }
      event "Autoscale": Value Change {
        n540 = event-data() -> ("NewVal"=w871:bool)  [unwired: 6 out]
        n541 = flat-sequence {
          tunnel: w872 -> [w885]
          tunnel: w871 -> [w874]
          tunnel: [w876] -> w870
          tunnel: [w875] -> w869
          tunnel: w868 -> [w875]
          tunnel: [w874] -> w867
          tunnel: [w873] -> w866
          tunnel: w870 -> [w920]
          tunnel: w869 -> [w914]
          tunnel: w867 -> [w913]
          tunnel: w866 -> [w912]
          frame #0 {
            n542 = local read "ScaleAxis"() -> (w876:u16)
            n543 = Select(t=u8 2 ("X Scale.Scale Fit"), s=w874, f=u8 0 ("X Scale.Scale Fit")) -> (s? t:f=w882:u8)
            n544 = local read "Maximum"() -> (w879:dbl)
            n545 = local read "Minimum"() -> (w878:dbl)
            n546 = Select(t=u8 2 ("X Scale.Scale Fit"), s=w874, f=u8 0 ("X Scale.Scale Fit")) -> (s? t:f=w877:u8)
            n547 = case shown="False" w874 {
              tunnel: w876 -> [w889 _]
              tunnel: w879 -> [w888 _]
              tunnel: w878 -> [w887 _]
              tunnel: w885 -> [w886 _]
              frame False {
                n548 = case shown="0, Default" w889 {
                  tunnel: w886 -> [w892 w896 w900]
                  tunnel: w888 -> [w891 w894 w898]
                  tunnel: w887 -> [w890 w893 w897]
                  frame 0, Default {
                    n549 = property class="WFGraph"(reference=w892, "XScale.Maximum"=w891, "XScale.Minimum"=w890) -> ()  [unwired: 1 in, 2 out]
                  }
                  frame 1 {
                    n550 = property class="WFGraph"(reference=w896, "ActYScl"=0 ("Active Y Scale"), "YScale.Maximum"=w894, "YScale.Minimum"=w893) -> ()  [unwired: 1 in, 2 out]
                  }
                  frame 2 {
                    n551 = property class="WFGraph"(reference=w900, "ActYScl"=1 ("Active Y Scale"), "YScale.Maximum"=w898, "YScale.Minimum"=w897) -> ()  [unwired: 1 in, 2 out]
                  }
                }
              }
              frame True {
              }
            }
            n552 = property on="Maximum" class="DigNum (strict)"("Disabled"=w877) -> ()  [unwired: 2 in, 2 out]
            n553 = property on="Minimum" class="DigNum (strict)"("Disabled"=w877) -> ()  [unwired: 2 in, 2 out]
            n554 = case shown="1" w876 {
              tunnel: w882 -> [w902 w906 w909]
              tunnel: w885 -> [w903 w907 w911]
              tunnel: ["ScaleFitX" ("Label Name") "ScaleFitY" ("Label Name") "ScaleFitY 2" ("Label Name")] -> w873
              frame 0, Default {
                n555 = property class="WFGraph"(reference=w903, "XScale.ScaleFit"=w902) -> ()  [unwired: 1 in, 2 out]
              }
              frame 1 {
                n556 = property class="WFGraph"(reference=w907, "ActYScl"=0 ("Active Y Scale"), "YScale.ScaleFit"=w906) -> ()  [unwired: 1 in, 2 out]
              }
              frame 2 {
                n557 = property class="WFGraph"(reference=w911, "ActYScl"=1 ("Active Y Scale"), "YScale.ScaleFit"=w909) -> ()  [unwired: 1 in, 2 out]
              }
            }
          }
          frame #1 {
            n558 = call "CRYGet Boolean Reference.vi"("Label Name"=w912, "VI Refnum"=w914) -> ("Boolean Ref"=w919:refnum<vi>, "VI Refnum Out"=w918:refnum<vi>)  [unwired: 7 in, 1 out]
            n559 = case shown="0, Default" w920 {
              tunnel: w914 -> [w921 _]
              frame 0, Default {
                n560 = call "CRYGet Boolean Reference.vi"("Label Name"="ScaleRange", "VI Refnum"=w921) -> ("Boolean Ref"=w923:refnum<vi>)  [unwired: 7 in, 2 out]
                n561 = property class="Bool"(reference=w923, "Val(Sgnl)"=TRUE) -> ()  [unwired: 1 in, 2 out]
              }
              frame 1 {
              }
            }
            n562 = property class="Bool"(reference=w919, "Value"=w913) -> (error out=w915:errorcluster)  [unwired: 1 in, 1 out]
            n563 = call "CRYGet Boolean Reference.vi"("Label Name"="ToolbarUpdate", "VI Refnum"=w918) -> ("Boolean Ref"=w916:refnum<vi>)  [unwired: 7 in, 2 out]
            n564 = property class="Bool"(reference=w916, error in=w915, "Val(Sgnl)"=w913) -> ()  [unwired: 2 out]
          }
        }
      }
      event "Minimum": Value Change {
        n565 = event-data() -> ("NewVal"=w927:dbl)  [unwired: 6 out]
        n566 = local write "Minimum"(w927) -> ()
        n567 = local read "ScaleAxis"() -> (w926:u16)
        n568 = case shown="0, Default" w926 {
          tunnel: w927 -> [w931 w939 w941]
          tunnel: w928 -> [w930 w940 w943]
          tunnel: w925 -> [w929 _ _]
          frame 0, Default {
            n569 = flat-sequence {
              tunnel: w931 -> [w933]
              tunnel: w930 -> [w932]
              tunnel: w929 -> [w934]
              frame #0 {
                n570 = property class="WFGraph"(reference=w932, "XScale.Minimum"=w933) -> ()  [unwired: 1 in, 2 out]
              }
              frame #1 {
                n571 = call "CRYGet Boolean Reference.vi"("Label Name"="ScaleRange", "VI Refnum"=w934) -> ("Boolean Ref"=w936:refnum<vi>)  [unwired: 7 in, 2 out]
                n572 = property class="Bool"(reference=w936, "Val(Sgnl)"=TRUE) -> ()  [unwired: 1 in, 2 out]
              }
            }
          }
          frame 1 {
            n573 = property class="WFGraph"(reference=w940, "ActYScl"=0 ("Active Y Scale"), "YScale.Minimum"=w939) -> ()  [unwired: 1 in, 2 out]
          }
          frame 2 {
            n574 = property class="WFGraph"(reference=w943, "ActYScl"=1 ("Active Y Scale"), "YScale.Minimum"=w941) -> ()  [unwired: 1 in, 2 out]
          }
        }
      }
      event "Maximum": Value Change {
        n575 = event-data() -> ("NewVal"=w946:dbl)  [unwired: 6 out]
        n576 = local write "Maximum"(w946) -> ()
        n577 = local read "ScaleAxis"() -> (w945:u16)
        n578 = case shown="0, Default" w945 {
          tunnel: w946 -> [w950 w958 w960]
          tunnel: w947 -> [w949 w959 w962]
          tunnel: w944 -> [w948 _ _]
          frame 0, Default {
            n579 = flat-sequence {
              tunnel: w950 -> [w952]
              tunnel: w949 -> [w951]
              tunnel: w948 -> [w953]
              frame #0 {
                n580 = property class="WFGraph"(reference=w951, "XScale.Maximum"=w952) -> ()  [unwired: 1 in, 2 out]
              }
              frame #1 {
                n581 = call "CRYGet Boolean Reference.vi"("Label Name"="ScaleRange", "VI Refnum"=w953) -> ("Boolean Ref"=w955:refnum<vi>)  [unwired: 7 in, 2 out]
                n582 = property class="Bool"(reference=w955, "Val(Sgnl)"=TRUE) -> ()  [unwired: 1 in, 2 out]
              }
            }
          }
          frame 1 {
            n583 = property class="WFGraph"(reference=w959, "ActYScl"=0 ("Active Y Scale"), "YScale.Maximum"=w958) -> ()  [unwired: 1 in, 2 out]
          }
          frame 2 {
            n584 = property class="WFGraph"(reference=w962, "ActYScl"=1 ("Active Y Scale"), "YScale.Maximum"=w960) -> ()  [unwired: 1 in, 2 out]
          }
        }
      }
      event "Show Cursors": Value Change {
        n585 = event-data() -> ("NewVal"=w963:bool)  [unwired: 6 out]
        n586 = local write "Show Cursors"(w963) -> ()
        n587 = Select(t=0, s=w963, f=2) -> (s? t:f=w969:i32)
        n588 = call "CRYGet Boolean Reference.vi"("Label Name"="CursorShow", "VI Refnum"=w966) -> ("Boolean Ref"=w964:refnum<vi>)  [unwired: 7 in, 2 out]
        n589 = property on="Cursor Tab" class="TabCtl (strict)"("DisabledEnum"=w969) -> ()  [unwired: 2 in, 2 out]
        n590 = property class="Bool"(reference=w964, "Val(Sgnl)"=w963) -> ()  [unwired: 1 in, 2 out]
      }
      event "Cursor Items": Value Change {
        n591 = event-data() -> ("NewVal"=w970:u16)  [unwired: 6 out]
        n592 = flat-sequence {
          tunnel: [w977] -> w972
          tunnel: w972 -> [w982]
          tunnel: w970 -> [w980]
          tunnel: w971 -> [w981]
          frame #0 {
            n593 = local read "CursorLineWidth"() -> (w975:string)
            n594 = local read "CursorPointStyle"() -> (w974:string)
            n595 = local read "CursorLineStyle"() -> (w976:string)
            n596 = control-ref of="This VI"() -> (w977:refnum<vi>)
            n597 = local read "CursorStyle"() -> (w973:string)
            n598 = To Variant(anything=FALSE) -> (Variant=w979:variant)
            n599 = invoke class="VI" method="Ctrl Val.Set"(reference=w977, "Control Name"=w976, "Value"=w979) -> ()  [unwired: 2 in, 5 out]
            n600 = invoke class="VI" method="Ctrl Val.Set"(reference=w977, "Control Name"=w975, "Value"=w979) -> ()  [unwired: 2 in, 5 out]
            n601 = invoke class="VI" method="Ctrl Val.Set"(reference=w977, "Control Name"=w974, "Value"=w979) -> ()  [unwired: 2 in, 5 out]
            n602 = invoke class="VI" method="Ctrl Val.Set"(reference=w977, "Control Name"=w973, "Value"=w979) -> ()  [unwired: 2 in, 5 out]
          }
          frame #1 {
            n603 = call "CRYSet Cursor Infor.vi"("This VI"=w982, "Active Cursor"=w980, "Graph Type"="WAVE", "Wave Graph Ref"=w981, "Property Set?"=TRUE) -> ("Cursor Color"=w983:u32, "CursorLineStyle"=w986:string, "CursorLineWidth"=w987:string, "CursorPointStyle"=w988:string, "CursorStyle"=w989:string)  [unwired: 17 in, 1 out]
            n604 = local write "CursorLineWidth"(w987) -> ()
            n605 = local write "Cursor color"(w983) -> ()
            n606 = local write "CursorLineStyle"(w986) -> ()
            n607 = local write "CursorPointStyle"(w988) -> ()
            n608 = local write "CursorStyle"(w989) -> ()
          }
        }
      }
      event "CursorLineStyle0", "CursorLineStyle1", "CursorLineStyle2", "CursorLineStyle3", "CursorLineStyle4": Value Change {
        n609 = event-data() -> ("CtlRef"=w990:refnum<vi>)  [unwired: 6 out]
        n610 = local read "CursorLineStyle"() -> (w991:string)
        n611 = property class="Bool (strict)"(reference=w990) -> ("Label.Text"=w994:string)  [unwired: 1 in, 2 out]
        n612 = Equal?(x=w994, y=w991) -> (x = y?=w993:bool)
        n613 = case shown="False" w993 {
          tunnel: w994 -> [w995 w1007]
          tunnel: w991 -> [w1005 _]
          tunnel: w992 -> [w996 _]
          frame False {
            n614 = control-ref of="This VI"() -> (w1006:refnum<vi>)
            n615 = Match Pattern(string=w995, regular expression="CursorLineStyle") -> (after substring=w998:string)  [unwired: 4 out]
            n616 = To Variant(anything=TRUE) -> (Variant=w1003:variant)
            n617 = Decimal String To Number(string=w998) -> (number=w997:i32)  [unwired: 3 out]
            n618 = invoke class="VI" method="Ctrl Val.Set"(reference=w1006, "Control Name"=w995, "Value"=w1003) -> (reference out=w1004:refnum<vi>)  [unwired: 2 in, 4 out]
            n619 = local write "CursorLineStyle"(w995) -> ()
            n620 = property class="WFGraph"(reference=w996, "Cursor.LineStyle"=w997) -> ()  [unwired: 1 in, 2 out]
            n621 = To Variant(anything=FALSE) -> (Variant=w1001:variant)
            n622 = invoke class="VI" method="Ctrl Val.Set"(reference=w1004, "Control Name"=w1005, "Value"=w1001) -> ()  [unwired: 2 in, 5 out]
          }
          frame True {
            n623 = control-ref of="This VI"() -> (w1010:refnum<vi>)
            n624 = To Variant(anything=TRUE) -> (Variant=w1009:variant)
            n625 = invoke class="VI" method="Ctrl Val.Set"(reference=w1010, "Control Name"=w1007, "Value"=w1009) -> ()  [unwired: 2 in, 5 out]
          }
        }
      }
      event "CursorLineWidth0", "CursorLineWidth1", "CursorLineWidth2", "CursorLineWidth3", "CursorLineWidth4", "CursorLineWidth5": Value Change {
        n626 = event-data() -> ("CtlRef"=w1011:refnum<vi>)  [unwired: 6 out]
        n627 = local read "CursorLineWidth"() -> (w1012:string)
        n628 = property class="Bool (strict)"(reference=w1011) -> ("Label.Text"=w1015:string)  [unwired: 1 in, 2 out]
        n629 = Equal?(x=w1015, y=w1012) -> (x = y?=w1014:bool)
        n630 = case shown="False" w1014 {
          tunnel: w1015 -> [w1016 w1028]
          tunnel: w1012 -> [w1026 _]
          tunnel: w1013 -> [w1017 _]
          frame False {
            n631 = control-ref of="This VI"() -> (w1027:refnum<vi>)
            n632 = Match Pattern(string=w1016, regular expression="CursorLineWidth") -> (after substring=w1019:string)  [unwired: 4 out]
            n633 = To Variant(anything=TRUE) -> (Variant=w1024:variant)
            n634 = Decimal String To Number(string=w1019) -> (number=w1020:i32)  [unwired: 3 out]
            n635 = invoke class="VI" method="Ctrl Val.Set"(reference=w1027, "Control Name"=w1016, "Value"=w1024) -> (reference out=w1025:refnum<vi>)  [unwired: 2 in, 4 out]
            n636 = local write "CursorLineWidth"(w1016) -> ()
            n637 = property class="WFGraph"(reference=w1017, "Cursor.LineWidth"=w1020) -> ()  [unwired: 1 in, 2 out]
            n638 = To Variant(anything=FALSE) -> (Variant=w1022:variant)
            n639 = invoke class="VI" method="Ctrl Val.Set"(reference=w1025, "Control Name"=w1026, "Value"=w1022) -> ()  [unwired: 2 in, 5 out]
          }
          frame True {
            n640 = control-ref of="This VI"() -> (w1031:refnum<vi>)
            n641 = To Variant(anything=TRUE) -> (Variant=w1030:variant)
            n642 = invoke class="VI" method="Ctrl Val.Set"(reference=w1031, "Control Name"=w1028, "Value"=w1030) -> ()  [unwired: 2 in, 5 out]
          }
        }
      }
      event "CursorPointStyle0", "CursorPointStyle1", "CursorPointStyle2", "CursorPointStyle3", "CursorPointStyle4", "CursorPointStyle5", "CursorPointStyle6", "CursorPointStyle7", "CursorPointStyle8", "CursorPointStyle10", "CursorPointStyle9", "CursorPointStyle11", "CursorPointStyle12", "CursorPointStyle13", "CursorPointStyle14", "CursorPointStyle15", "CursorPointStyle16": Value Change {
        n643 = event-data() -> ("CtlRef"=w1033:refnum<vi>)  [unwired: 6 out]
        n644 = local read "CursorPointStyle"() -> (w1032:string)
        n645 = property class="Bool (strict)"(reference=w1033) -> ("Label.Text"=w1036:string)  [unwired: 1 in, 2 out]
        n646 = Equal?(x=w1036, y=w1032) -> (x = y?=w1035:bool)
        n647 = case shown="False" w1035 {
          tunnel: w1036 -> [w1037 w1049]
          tunnel: w1032 -> [w1047 _]
          tunnel: w1034 -> [w1038 _]
          frame False {
            n648 = control-ref of="This VI"() -> (w1048:refnum<vi>)
            n649 = To Variant(anything=TRUE) -> (Variant=w1045:variant)
            n650 = Match Pattern(string=w1037, regular expression="CursorPointStyle") -> (after substring=w1040:string)  [unwired: 4 out]
            n651 = invoke class="VI" method="Ctrl Val.Set"(reference=w1048, "Control Name"=w1037, "Value"=w1045) -> (reference out=w1046:refnum<vi>)  [unwired: 2 in, 4 out]
            n652 = Decimal String To Number(string=w1040) -> (number=w1041:i32)  [unwired: 3 out]
            n653 = local write "CursorPointStyle"(w1037) -> ()
            n654 = property class="WFGraph"(reference=w1038, "Cursor.Cursor Point Style"=w1041) -> ()  [unwired: 1 in, 2 out]
            n655 = To Variant(anything=FALSE) -> (Variant=w1043:variant)
            n656 = invoke class="VI" method="Ctrl Val.Set"(reference=w1046, "Control Name"=w1047, "Value"=w1043) -> ()  [unwired: 2 in, 5 out]
          }
          frame True {
            n657 = control-ref of="This VI"() -> (w1052:refnum<vi>)
            n658 = To Variant(anything=TRUE) -> (Variant=w1051:variant)
            n659 = invoke class="VI" method="Ctrl Val.Set"(reference=w1052, "Control Name"=w1049, "Value"=w1051) -> ()  [unwired: 2 in, 5 out]
          }
        }
      }
      event "CursorStyle0", "CursorStyle1", "CursorStyle2", "CursorStyle3", "CursorStyle6", "CursorStyle7", "CursorStyle5", "CursorStyle4", "CursorStyle8": Value Change {
        n660 = event-data() -> ("CtlRef"=w1054:refnum<vi>)  [unwired: 6 out]
        n661 = local read "CursorStyle"() -> (w1053:string)
        n662 = property class="Bool (strict)"(reference=w1054) -> ("Label.Text"=w1057:string)  [unwired: 1 in, 2 out]
        n663 = Equal?(x=w1057, y=w1053) -> (x = y?=w1056:bool)
        n664 = case shown="False" w1056 {
          tunnel: w1057 -> [w1058 w1070]
          tunnel: w1053 -> [w1068 _]
          tunnel: w1055 -> [w1059 _]
          frame False {
            n665 = control-ref of="This VI"() -> (w1069:refnum<vi>)
            n666 = To Variant(anything=TRUE) -> (Variant=w1066:variant)
            n667 = Match Pattern(string=w1058, regular expression="CursorStyle") -> (after substring=w1061:string)  [unwired: 4 out]
            n668 = invoke class="VI" method="Ctrl Val.Set"(reference=w1069, "Control Name"=w1058, "Value"=w1066) -> (reference out=w1067:refnum<vi>)  [unwired: 2 in, 4 out]
            n669 = Decimal String To Number(string=w1061) -> (number=w1062:i32)  [unwired: 3 out]
            n670 = local write "CursorStyle"(w1058) -> ()
            n671 = property class="WFGraph"(reference=w1059, "Cursor.Cursor Style"=w1062) -> ()  [unwired: 1 in, 2 out]
            n672 = To Variant(anything=FALSE) -> (Variant=w1064:variant)
            n673 = invoke class="VI" method="Ctrl Val.Set"(reference=w1067, "Control Name"=w1068, "Value"=w1064) -> ()  [unwired: 2 in, 5 out]
          }
          frame True {
            n674 = control-ref of="This VI"() -> (w1073:refnum<vi>)
            n675 = To Variant(anything=TRUE) -> (Variant=w1072:variant)
            n676 = invoke class="VI" method="Ctrl Val.Set"(reference=w1073, "Control Name"=w1070, "Value"=w1072) -> ()  [unwired: 2 in, 5 out]
          }
        }
      }
      event "Cursor color": Value Change {
        n677 = event-data() -> ("NewVal"=w1080:u32)  [unwired: 6 out]
        n678 = property class="WFGraph"(reference=w1078) -> (reference out=w1077:refnum<vi>, "Active Cursor"=w1075:u32)  [unwired: 1 in, 1 out]
        n679 = local read "Cursor Items"() -> (w1081:u16)
        n680 = local write "Cursor color"(w1080) -> ()
        n681 = property class="WFGraph"(reference=w1077, "Active Cursor"=w1081, "Cursor.Cursor Color"=w1080) -> (reference out=w1076:refnum<vi>)  [unwired: 1 in, 1 out]
        n682 = property class="WFGraph"(reference=w1076, "Active Cursor"=w1075) -> (reference out=w1074:refnum<vi>)  [unwired: 1 in, 1 out]
        n683 = flat-sequence {
          tunnel: w1079 -> [w1082]
          tunnel: w1074 -> [_]
          frame #0 {
            n684 = call "CRYGet Boolean Reference.vi"("Label Name"="CursorColor" ("Control Name"), "VI Refnum"=w1082) -> ("Boolean Ref"=w1084:refnum<vi>)  [unwired: 7 in, 2 out]
            n685 = property class="Bool"(reference=w1084, "Val(Sgnl)"=TRUE ("Visible")) -> ()  [unwired: 1 in, 2 out]
          }
        }
      }
      event "Linked to plot:": Value Change {
        n686 = event-data() -> ("NewVal"=w1097:u16)  [unwired: 6 out]
        n687 = local write "Linked to plot:"(w1097) -> ()
        n688 = local read "Cursor Items"() -> (w1088:u16)
        n689 = property class="WFGraph"(reference=w1098, "Active Cursor"=w1088, "Cursor.Cursor Plot"=w1097) -> (reference out=w1089:refnum<vi>)  [unwired: 1 in, 1 out]
        n690 = property class="Tbl"(reference=w1087) -> ("Value"=w1090:string[][])  [unwired: 1 in, 2 out]
        n691 = Index Array(array=w1090, index (row)=w1088) -> (element=w1091:string[])  [unwired: 1 in]
        n692 = Index Array(array=w1091, index=1) -> (element=w1093:string)
        n693 = Match Pattern(string=w1093, regular expression=":" ("string")) -> (after substring=w1096:string, offset past match=w1095:i32)  [unwired: 1 in, 2 out]
        n694 = case shown="1.." w1095 {
          tunnel: w1096 -> [w1104 _]
          tunnel: w1089 -> [w1102 _]
          tunnel: w1088 -> [w1101 _]
          tunnel: w1086 -> [w1099 _]
          frame 1.. {
            n695 = Fract/Exp String To Number(string=w1104) -> (number=w1103:dbl)  [unwired: 3 in, 1 out]
            n696 = property class="WFGraph"(reference=w1102, "Active Cursor"=w1101, "Cursor.Cursor X"=w1103) -> (reference out=w1100:refnum<vi>)  [unwired: 1 in, 1 out]
            n697 = flat-sequence {
              tunnel: w1100 -> [_]
              tunnel: w1099 -> [w1107]
              frame #0 {
                n698 = call "CRYGet Boolean Reference.vi"("Label Name"="CursorPlot", "VI Refnum"=w1107) -> ("Boolean Ref"=w1106:refnum<vi>)  [unwired: 7 in, 2 out]
                n699 = property class="Bool"(reference=w1106, "Val(Sgnl)"=TRUE) -> ()  [unwired: 1 in, 2 out]
              }
            }
          }
          frame ..0 {
          }
        }
      }
      event "Link Cursors": Value Change {
        n700 = event-data() -> ("NewVal"=w1109:bool)  [unwired: 6 out]
        n701 = local write "Link Cursors"(w1109) -> ()
      }
    }
  }
